vi "DriveSplinePathPlanner.vi"(3 "error in (no error)":errorcluster, 4 "DrivePathPlanParams":T2={"max_velocity (in/s)"=72.0, "max_acceleration (in/s^2)"=20.0, "max_jerk (in/s^3)"=60.0, "dt(ms)"=10, "sample_count"=1000, "wheelbase_width (in)"=24.0} {"dt(ms)" items=["TrajectoryDuration_0ms"=0, "TrajectoryDuration_5ms"=5, "TrajectoryDuration_10ms"=10, "TrajectoryDuration_20ms"=20, "TrajectoryDuration_30ms"=30, "TrajectoryDuration_40ms"=40, "TrajectoryDuration_50ms"=50, "TrajectoryDuration_100ms"=100]}, 5 "path":T5[](array[typedef])=[{"x"=12.0, "y"=150.0, "angle"=0.0}, {"x"=24.0, "y"=150.0, "angle"=0.0}, {"x"=175.0, "y"=275.0, "angle"=0.0}, {"x"=235.0, "y"=200.0, "angle"=90.0}, {"x"=235.0, "y"=125.0, "angle"=90.0}, {"x"=290.0, "y"=65.0, "angle"=0.0}]) -> (0 "error out":errorcluster, 1 "RightTrajectory":T1[](array[typedef]), 2 "LeftTrajectory":T1[](array[typedef]))   [LabVIEW 2017]
uses:
  Pathfinder/Pathfinder-LabVIEW/Pathfinder-Lib/VIs/Waypoint.ctl
  PathPlannerSupport/TypeDefs/DrivePathfinderParams.ctl
  <vilib>/Rock Robotics/WPI/ThirdParty/Phoenix-LabVIEW/Motor Controller/Controls/CTRE_Phoenix_MotorControl_TrajectoryPointTimeDur.ctl
  Pathfinder/Pathfinder-LabVIEW/Pathfinder-Lib/VIs/Segment.ctl
  Pathfinder/Pathfinder-LabVIEW/Pathfinder-Lib/Pathfinder.lvlib
panel:
  in  "Tab Control":enum32{"Primary Path", "Tank Position"}(tab)
  out "Path":T4(graph)=[{"position"=2.9411764705882357e-05, "velocity"=0.005882352941176471, "acceleration"=0.5882352941176471, "jerk"=58.82352941176471, "heading"=0.0}, {"position"=0.00014705882352941178, "velocity"=0.01764705882352941, "acceleration"=1.1764705882352942, "jerk"=58.82352941176471, "heading"=0.0}, {"position"=0.0004117647058823529, "velocity"=0.03529411764705882, "acceleration"=1.7647058823529411, "jerk"=58.823529411764696, "heading"=0.0}, {"position"=0.0008823529411764706, "velocity"=0.0588235294117647, "acceleration"=2.3529411764705874, "jerk"=58.82352941176463, "heading"=0.0}, {"position"=0.0016176470588235292, "velocity"=0.08823529411764705, "acceleration"=2.941176470588235, "jerk"=58.82352941176476, "heading"=0.0}, {"position"=0.002676470588235294, "velocity"=0.12352941176470589, "acceleration"=3.5294117647058836, "jerk"=58.82352941176485, "heading"=0.0}, {"position"=0.00411764705882353, "velocity"=0.16470588235294117, "acceleration"=4.117647058823529, "jerk"=58.82352941176454, "heading"=0.0}, {"position"=0.006, "velocity"=0.21176470588235294, "acceleration"=4.705882352941177, "jerk"=58.82352941176476, "heading"=0.0}, {"position"=0.008382352941176471, "velocity"=0.2647058823529412, "acceleration"=5.294117647058824, "jerk"=58.82352941176476, "heading"=0.0}, {"position"=0.011323529411764706, "velocity"=0.3235294117647059, "acceleration"=5.882352941176472, "jerk"=58.82352941176476, "heading"=0.0}, {"position"=0.014882352941176472, "velocity"=0.38823529411764707, "acceleration"=6.470588235294117, "jerk"=58.8235294117645, "heading"=0.0}, {"position"=0.01911764705882353, "velocity"=0.4588235294117647, "acceleration"=7.058823529411762, "jerk"=58.8235294117645, "heading"=0.0}, {"position"=0.02408823529411765, "velocity"=0.5352941176470588, "acceleration"=7.647058823529412, "jerk"=58.82352941176503, "heading"=0.0}, {"position"=0.02985294117647059, "velocity"=0.6176470588235294, "acceleration"=8.235294117647063, "jerk"=58.823529411765115, "heading"=0.0}, {"position"=0.036470588235294116, "velocity"=0.7058823529411764, "acceleration"=8.823529411764696, "jerk"=58.82352941176325, "heading"=0.0}, {"position"=0.044, "velocity"=0.8, "acceleration"=9.411764705882364, "jerk"=58.823529411766806, "heading"=0.0}, {"position"=0.0525, "velocity"=0.8999999999999999, "acceleration"=9.999999999999986, "jerk"=58.82352941176219, "heading"=0.0}, {"position"=0.06202941176470588, "velocity"=1.0058823529411764, "acceleration"=10.588235294117654, "jerk"=58.823529411766806, "heading"=0.0}, {"position"=0.07264705882352941, "velocity"=1.1176470588235294, "acceleration"=11.176470588235299, "jerk"=58.8235294117645, "heading"=0.0}, {"position"=0.08441176470588235, "velocity"=1.2352941176470589, "acceleration"=11.764705882352944, "jerk"=58.8235294117645, "heading"=0.0}, {"position"=0.09738235294117648, "velocity"=1.3588235294117648, "acceleration"=12.352941176470589, "jerk"=58.8235294117645, "heading"=0.0}, {"position"=0.11161764705882353, "velocity"=1.488235294117647, "acceleration"=12.941176470588234, "jerk"=58.8235294117645, "heading"=0.0}, {"position"=0.1271764705882353, "velocity"=1.623529411764706, "acceleration"=13.5294117647059, "jerk"=58.82352941176663, "heading"=0.0}, {"position"=0.14411764705882354, "velocity"=1.7647058823529411, "acceleration"=14.1176470588235, "jerk"=58.823529411760056, "heading"=0.0}, {"position"=0.1625, "velocity"=1.9117647058823528, "acceleration"=14.705882352941169, "jerk"=58.823529411766806, "heading"=0.0}, {"position"=0.18238235294117647, "velocity"=2.064705882352941, "acceleration"=15.294117647058814, "jerk"=58.8235294117645, "heading"=0.0}, {"position"=0.2038235294117647, "velocity"=2.223529411764706, "acceleration"=15.882352941176503, "jerk"=58.82352941176894, "heading"=0.0}, {"position"=0.22688235294117648, "velocity"=2.388235294117647, "acceleration"=16.4705882352941, "jerk"=58.82352941175988, "heading"=0.0}, {"position"=0.25161764705882356, "velocity"=2.5588235294117645, "acceleration"=17.058823529411747, "jerk"=58.8235294117645, "heading"=0.0}, {"position"=0.2780882352941177, "velocity"=2.735294117647059, "acceleration"=17.647058823529438, "jerk"=58.823529411769115, "heading"=0.0}, {"position"=0.3063529411764706, "velocity"=2.9176470588235297, "acceleration"=18.235294117647083, "jerk"=58.8235294117645, "heading"=0.0}, {"position"=0.33647058823529413, "velocity"=3.1058823529411765, "acceleration"=18.82352941176468, "jerk"=58.82352941175988, "heading"=0.0}, {"position"=0.3685, "velocity"=3.3000000000000003, "acceleration"=19.411764705882373, "jerk"=58.823529411769115, "heading"=0.0}, {"position"=0.40249999999999997, "velocity"=3.4999999999999996, "acceleration"=19.99999999999993, "jerk"=58.823529411755615, "heading"=0.0}, {"position"=0.43849999999999995, "velocity"=3.6999999999999997, "acceleration"=20.000000000000018, "jerk"=8.881784197001252e-12, "heading"=0.0}, {"position"=0.4764999999999999, "velocity"=3.8999999999999995, "acceleration"=19.99999999999997, "jerk"=-4.618527782440651e-12, "heading"=0.0}, {"position"=0.5165, "velocity"=4.1, "acceleration"=20.000000000000018, "jerk"=4.618527782440651e-12, "heading"=0.0}, {"position"=0.5585, "velocity"=4.3, "acceleration"=20.000000000000018, "jerk"=0.0, "heading"=0.0}, {"position"=0.6025, "velocity"=4.5, "acceleration"=20.000000000000018, "jerk"=0.0, "heading"=0.0}, {"position"=0.6485000000000001, "velocity"=4.7, "acceleration"=20.000000000000018, "jerk"=0.0, "heading"=0.0}, {"position"=0.6965000000000001, "velocity"=4.9, "acceleration"=20.000000000000018, "jerk"=0.0, "heading"=0.0}, {"position"=0.7465000000000002, "velocity"=5.1, "acceleration"=19.99999999999993, "jerk"=-8.881784197001252e-12, "heading"=0.0}, {"position"=0.7985000000000002, "velocity"=5.3, "acceleration"=20.000000000000018, "jerk"=8.881784197001252e-12, "heading"=0.0}, {"position"=0.8525000000000003, "velocity"=5.5, "acceleration"=20.000000000000018, "jerk"=0.0, "heading"=0.0}, {"position"=0.9085000000000003, "velocity"=5.700000000000001, "acceleration"=20.000000000000107, "jerk"=8.881784197001252e-12, "heading"=0.0}, {"position"=0.9665000000000004, "velocity"=5.9, "acceleration"=19.99999999999993, "jerk"=-1.7763568394002505e-11, "heading"=0.0}, {"position"=1.0265000000000004, "velocity"=6.1000000000000005, "acceleration"=20.000000000000018, "jerk"=8.881784197001252e-12, "heading"=0.0}, {"position"=1.0885000000000005, "velocity"=6.300000000000001, "acceleration"=20.000000000000018, "jerk"=0.0, "heading"=0.0}, {"position"=1.1525000000000005, "velocity"=6.500000000000001, "acceleration"=20.000000000000018, "jerk"=0.0, "heading"=0.0}, {"position"=1.2185000000000006, "velocity"=6.7, "acceleration"=19.99999999999993, "jerk"=-8.881784197001252e-12, "heading"=0.0}, {"position"=1.2865000000000006, "velocity"=6.8999999999999995, "acceleration"=19.99999999999993, "jerk"=0.0, "heading"=0.0}, {"position"=1.3565000000000007, "velocity"=7.1, "acceleration"=20.000000000000018, "jerk"=8.881784197001252e-12, "heading"=0.0}, {"position"=1.4285000000000008, "velocity"=7.3, "acceleration"=20.000000000000018, "jerk"=0.0, "heading"=0.0}, {"position"=1.5025000000000008, "velocity"=7.499999999999999, "acceleration"=19.99999999999993, "jerk"=-8.881784197001252e-12, "heading"=0.0}, {"position"=1.578500000000001, "velocity"=7.699999999999999, "acceleration"=20.000000000000018, "jerk"=8.881784197001252e-12, "heading"=0.0}, {"position"=1.656500000000001, "velocity"=7.9, "acceleration"=20.000000000000107, "jerk"=8.881784197001252e-12, "heading"=0.0}, {"position"=1.736500000000001, "velocity"=8.1, "acceleration"=19.99999999999993, "jerk"=-1.7763568394002505e-11, "heading"=0.0}, {"position"=1.8185000000000011, "velocity"=8.299999999999999, "acceleration"=19.99999999999993, "jerk"=0.0, "heading"=0.0}, {"position"=1.9025000000000012, "velocity"=8.5, "acceleration"=20.000000000000107, "jerk"=1.7763568394002505e-11, "heading"=0.0}, {"position"=1.9885000000000013, "velocity"=8.7, "acceleration"=19.99999999999993, "jerk"=-1.7763568394002505e-11, "heading"=0.0}, {"position"=2.076500000000001, "velocity"=8.899999999999999, "acceleration"=19.99999999999993, "jerk"=0.0, "heading"=0.0}, {"position"=2.166500000000001, "velocity"=9.1, "acceleration"=20.000000000000107, "jerk"=1.7763568394002505e-11, "heading"=0.0}, {"position"=2.258500000000001, "velocity"=9.299999999999999, "acceleration"=19.99999999999993, "jerk"=-1.7763568394002505e-11, "heading"=0.0}, {"position"=2.352500000000001, "velocity"=9.499999999999998, "acceleration"=19.99999999999993, "jerk"=0.0, "heading"=0.0}, {"position"=2.448500000000001, "velocity"=9.7, "acceleration"=20.000000000000107, "jerk"=1.7763568394002505e-11, "heading"=0.0}, {"position"=2.546500000000001, "velocity"=9.899999999999999, "acceleration"=19.99999999999993, "jerk"=-1.7763568394002505e-11, "heading"=0.0}, {"position"=2.646500000000001, "velocity"=10.1, "acceleration"=20.000000000000107, "jerk"=1.7763568394002505e-11, "heading"=0.0}, {"position"=2.748500000000001, "velocity"=10.299999999999999, "acceleration"=19.99999999999993, "jerk"=-1.7763568394002505e-11, "heading"=0.0}, {"position"=2.852500000000001, "velocity"=10.499999999999998, "acceleration"=19.99999999999993, "jerk"=0.0, "heading"=0.0}, {"position"=2.958500000000001, "velocity"=10.7, "acceleration"=20.000000000000107, "jerk"=1.7763568394002505e-11, "heading"=0.0}, {"position"=3.066500000000001, "velocity"=10.899999999999999, "acceleration"=19.99999999999993, "jerk"=-1.7763568394002505e-11, "heading"=0.0}, {"position"=3.1765000000000008, "velocity"=11.099999999999998, "acceleration"=19.99999999999993, "jerk"=0.0, "heading"=0.0}, {"position"=3.288500000000001, "velocity"=11.3, "acceleration"=20.000000000000284, "jerk"=3.552713678800501e-11, "heading"=0.0}, {"position"=3.4025000000000007, "velocity"=11.5, "acceleration"=19.99999999999993, "jerk"=-3.552713678800501e-11, "heading"=0.0}, {"position"=3.518500000000001, "velocity"=11.700000000000001, "acceleration"=20.000000000000107, "jerk"=1.7763568394002505e-11, "heading"=0.0}, {"position"=3.6365000000000007, "velocity"=11.9, "acceleration"=19.99999999999993, "jerk"=-1.7763568394002505e-11, "heading"=0.0}, {"position"=3.756500000000001, "velocity"=12.1, "acceleration"=19.99999999999993, "jerk"=0.0, "heading"=0.0}, {"position"=3.8785000000000007, "velocity"=12.3, "acceleration"=20.000000000000107, "jerk"=1.7763568394002505e-11, "heading"=0.0}, {"position"=4.0025, "velocity"=12.5, "acceleration"=19.99999999999993, "jerk"=-1.7763568394002505e-11, "heading"=0.0}, {"position"=4.128500000000001, "velocity"=12.7, "acceleration"=19.99999999999993, "jerk"=0.0, "heading"=0.0}, {"position"=4.256500000000001, "velocity"=12.9, "acceleration"=20.000000000000107, "jerk"=1.7763568394002505e-11, "heading"=0.0}, {"position"=4.386500000000001, "velocity"=13.1, "acceleration"=19.99999999999993, "jerk"=-1.7763568394002505e-11, "heading"=0.0}, {"position"=4.5185, "velocity"=13.3, "acceleration"=20.000000000000107, "jerk"=1.7763568394002505e-11, "heading"=0.0}, {"position"=4.652500000000001, "velocity"=13.5, "acceleration"=19.99999999999993, "jerk"=-1.7763568394002505e-11, "heading"=0.0}, {"position"=4.788500000000001, "velocity"=13.7, "acceleration"=19.99999999999993, "jerk"=0.0, "heading"=0.0}, {"position"=4.926500000000001, "velocity"=13.9, "acceleration"=20.000000000000107, "jerk"=1.7763568394002505e-11, "heading"=0.0}, {"position"=5.0665000000000004, "velocity"=14.1, "acceleration"=19.99999999999993, "jerk"=-1.7763568394002505e-11, "heading"=0.0}, {"position"=5.208500000000001, "velocity"=14.3, "acceleration"=20.000000000000107, "jerk"=1.7763568394002505e-11, "heading"=0.0}, {"position"=5.352500000000001, "velocity"=14.5, "acceleration"=19.99999999999993, "jerk"=-1.7763568394002505e-11, "heading"=0.0}, {"position"=5.498500000000001, "velocity"=14.7, "acceleration"=19.99999999999993, "jerk"=0.0, "heading"=0.0}, {"position"=5.6465000000000005, "velocity"=14.9, "acceleration"=20.000000000000107, "jerk"=1.7763568394002505e-11, "heading"=0.0}, {"position"=5.796500000000001, "velocity"=15.1, "acceleration"=19.99999999999993, "jerk"=-1.7763568394002505e-11, "heading"=0.0}, {"position"=5.948500000000001, "velocity"=15.299999999999999, "acceleration"=19.99999999999993, "jerk"=0.0, "heading"=0.0}, {"position"=6.102500000000001, "velocity"=15.5, "acceleration"=20.000000000000107, "jerk"=1.7763568394002505e-11, "heading"=0.0}, {"position"=6.258500000000001, "velocity"=15.7, "acceleration"=19.99999999999993, "jerk"=-1.7763568394002505e-11, "heading"=0.0}, {"position"=6.416500000000001, "velocity"=15.900000000000002, "acceleration"=20.000000000000284, "jerk"=3.552713678800501e-11, "heading"=0.0}, {"position"=6.576500000000001, "velocity"=16.1, "acceleration"=19.99999999999993, "jerk"=-3.552713678800501e-11, "heading"=0.0}, {"position"=6.738500000000001, "velocity"=16.3, "acceleration"=19.99999999999993, "jerk"=0.0, "heading"=0.0}, {"position"=6.902500000000001, "velocity"=16.5, "acceleration"=19.99999999999993, "jerk"=0.0, "heading"=0.0}, {"position"=7.068500000000001, "velocity"=16.7, "acceleration"=19.99999999999993, "jerk"=0.0, "heading"=0.0}, {"position"=7.236500000000001, "velocity"=16.9, "acceleration"=19.99999999999993, "jerk"=0.0, "heading"=0.0}, {"position"=7.406500000000001, "velocity"=17.099999999999998, "acceleration"=19.99999999999993, "jerk"=0.0, "heading"=0.0}, {"position"=7.578500000000001, "velocity"=17.3, "acceleration"=20.000000000000284, "jerk"=3.552713678800501e-11, "heading"=0.0}, {"position"=7.752500000000001, "velocity"=17.5, "acceleration"=19.99999999999993, "jerk"=-3.552713678800501e-11, "heading"=0.0}, {"position"=7.928500000000001, "velocity"=17.7, "acceleration"=19.99999999999993, "jerk"=0.0, "heading"=0.0}, {"position"=8.106500000000002, "velocity"=17.9, "acceleration"=19.99999999999993, "jerk"=0.0, "heading"=0.0}, {"position"=8.286500000000002, "velocity"=18.1, "acceleration"=20.000000000000284, "jerk"=3.552713678800501e-11, "heading"=0.0}, {"position"=8.468500000000002, "velocity"=18.300000000000004, "acceleration"=20.000000000000284, "jerk"=0.0, "heading"=0.0}, {"position"=8.652500000000002, "velocity"=18.5, "acceleration"=19.999999999999574, "jerk"=-7.105427357601002e-11, "heading"=0.0}, {"position"=8.838500000000002, "velocity"=18.700000000000003, "acceleration"=20.000000000000284, "jerk"=7.105427357601002e-11, "heading"=0.0}, {"position"=9.026500000000002, "velocity"=18.900000000000002, "acceleration"=19.99999999999993, "jerk"=-3.552713678800501e-11, "heading"=0.0}, {"position"=9.216500000000002, "velocity"=19.1, "acceleration"=19.99999999999993, "jerk"=0.0, "heading"=0.0}, {"position"=9.408500000000002, "velocity"=19.3, "acceleration"=19.99999999999993, "jerk"=0.0, "heading"=0.0}, {"position"=9.602500000000003, "velocity"=19.500000000000004, "acceleration"=20.000000000000284, "jerk"=3.552713678800501e-11, "heading"=0.0}, {"position"=9.798500000000002, "velocity"=19.7, "acceleration"=19.999999999999574, "jerk"=-7.105427357601002e-11, "heading"=0.0}, {"position"=9.996500000000003, "velocity"=19.900000000000002, "acceleration"=20.000000000000284, "jerk"=7.105427357601002e-11, "heading"=0.0}, {"position"=10.196500000000002, "velocity"=20.1, "acceleration"=19.99999999999993, "jerk"=-3.552713678800501e-11, "heading"=0.0}, {"position"=10.398500000000002, "velocity"=20.3, "acceleration"=19.99999999999993, "jerk"=0.0, "heading"=0.0}, {"position"=10.602500000000003, "velocity"=20.5, "acceleration"=19.99999999999993, "jerk"=0.0, "heading"=0.0}, {"position"=10.808500000000002, "velocity"=20.700000000000003, "acceleration"=20.000000000000284, "jerk"=3.552713678800501e-11, "heading"=0.0}, {"position"=11.016500000000002, "velocity"=20.9, "acceleration"=19.999999999999574, "jerk"=-7.105427357601002e-11, "heading"=0.0}, {"position"=11.226500000000003, "velocity"=21.1, "acceleration"=20.000000000000284, "jerk"=7.105427357601002e-11, "heading"=0.0}, {"position"=11.438500000000003, "velocity"=21.3, "acceleration"=19.99999999999993, "jerk"=-3.552713678800501e-11, "heading"=0.0}, {"position"=11.652500000000003, "velocity"=21.500000000000004, "acceleration"=20.000000000000284, "jerk"=3.552713678800501e-11, "heading"=0.0}, {"position"=11.868500000000003, "velocity"=21.7, "acceleration"=19.999999999999574, "jerk"=-7.105427357601002e-11, "heading"=0.0}, {"position"=12.086500000000003, "velocity"=21.900000000000002, "acceleration"=20.000000000000284, "jerk"=7.105427357601002e-11, "heading"=359.8806943068728}, {"position"=12.306500000000003, "velocity"=22.1, "acceleration"=19.99999999999993, "jerk"=-3.552713678800501e-11, "heading"=0.026596597273722586}, {"position"=12.528500000000003, "velocity"=22.3, "acceleration"=19.99999999999993, "jerk"=0.0, "heading"=0.1743535565500996}, {"position"=12.752500000000003, "velocity"=22.5, "acceleration"=19.99999999999993, "jerk"=0.0, "heading"=0.32416768747403213}, {"position"=12.978500000000004, "velocity"=22.7, "acceleration"=19.99999999999993, "jerk"=0.0, "heading"=0.47603410075499847}, {"position"=13.206500000000004, "velocity"=22.9, "acceleration"=19.99999999999993, "jerk"=0.0, "heading"=0.6299618295768361}, {"position"=13.436500000000004, "velocity"=23.099999999999998, "acceleration"=19.99999999999993, "jerk"=0.0, "heading"=0.7859727327629965}, {"position"=13.668500000000003, "velocity"=23.3, "acceleration"=20.000000000000284, "jerk"=3.552713678800501e-11, "heading"=0.9440887403185972}, {"position"=13.902500000000003, "velocity"=23.499999999999996, "acceleration"=19.999999999999574, "jerk"=-7.105427357601002e-11, "heading"=1.1043318455056377}, {"position"=14.138500000000004, "velocity"=23.7, "acceleration"=20.000000000000284, "jerk"=7.105427357601002e-11, "heading"=1.2667240964869242}, {"position"=14.376500000000004, "velocity"=23.9, "acceleration"=19.99999999999993, "jerk"=-3.552713678800501e-11, "heading"=1.4312875875241853}, {"position"=14.616500000000004, "velocity"=24.1, "acceleration"=20.000000000000284, "jerk"=3.552713678800501e-11, "heading"=1.5980444497155757}, {"position"=14.858500000000003, "velocity"=24.299999999999997, "acceleration"=19.999999999999574, "jerk"=-7.105427357601002e-11, "heading"=1.7670168412578064}, {"position"=15.102500000000003, "velocity"=24.5, "acceleration"=20.000000000000284, "jerk"=7.105427357601002e-11, "heading"=1.938226937217854}, {"position"=15.348500000000003, "velocity"=24.7, "acceleration"=19.99999999999993, "jerk"=-3.552713678800501e-11, "heading"=2.111696918798984}, {"position"=15.596500000000002, "velocity"=24.9, "acceleration"=19.99999999999993, "jerk"=0.0, "heading"=2.2874489620858793}, {"position"=15.846500000000002, "velocity"=25.099999999999998, "acceleration"=19.99999999999993, "jerk"=0.0, "heading"=2.4655052262535966}, {"position"=16.0985, "velocity"=25.3, "acceleration"=20.000000000000284, "jerk"=3.552713678800501e-11, "heading"=2.6458878412247393}, {"position"=16.352500000000003, "velocity"=25.499999999999996, "acceleration"=19.999999999999574, "jerk"=-7.105427357601002e-11, "heading"=2.8286188947596687}, {"position"=16.608500000000003, "velocity"=25.7, "acceleration"=20.000000000000284, "jerk"=7.105427357601002e-11, "heading"=3.0137204189641817}, {"position"=16.866500000000002, "velocity"=25.9, "acceleration"=19.99999999999993, "jerk"=-3.552713678800501e-11, "heading"=3.2012143761994194}, {"position"=17.126500000000004, "velocity"=26.099999999999998, "acceleration"=19.99999999999993, "jerk"=0.0, "heading"=3.391122644378866}, {"position"=17.388500000000004, "velocity"=26.299999999999997, "acceleration"=19.99999999999993, "jerk"=0.0, "heading"=3.5834670016371466}, {"position"=17.652500000000003, "velocity"=26.5, "acceleration"=20.000000000000284, "jerk"=3.552713678800501e-11, "heading"=3.7782691103560753}, {"position"=17.9185, "velocity"=26.699999999999996, "acceleration"=19.999999999999574, "jerk"=-7.105427357601002e-11, "heading"=3.975550500533184}, {"position"=18.186500000000002, "velocity"=26.9, "acceleration"=20.000000000000284, "jerk"=7.105427357601002e-11, "heading"=4.175332552478496}, {"position"=18.456500000000002, "velocity"=27.1, "acceleration"=20.000000000000284, "jerk"=0.0, "heading"=4.377658335678091}, {"position"=18.7285, "velocity"=27.300000000000004, "acceleration"=20.000000000000284, "jerk"=0.0, "heading"=4.582559037811216}, {"position"=19.0025, "velocity"=27.5, "acceleration"=19.999999999999574, "jerk"=-7.105427357601002e-11, "heading"=4.7900277371429345}, {"position"=19.2785, "velocity"=27.700000000000003, "acceleration"=20.000000000000284, "jerk"=7.105427357601002e-11, "heading"=5.000085015447648}, {"position"=19.5565, "velocity"=27.900000000000002, "acceleration"=19.99999999999993, "jerk"=-3.552713678800501e-11, "heading"=5.212751205515084}, {"position"=19.8365, "velocity"=28.1, "acceleration"=19.99999999999993, "jerk"=0.0, "heading"=5.4280463694673555}, {"position"=20.1185, "velocity"=28.3, "acceleration"=19.99999999999993, "jerk"=0.0, "heading"=5.6460030928801945}, {"position"=20.4025, "velocity"=28.500000000000004, "acceleration"=20.000000000000284, "jerk"=3.552713678800501e-11, "heading"=5.8666951092504585}, {"position"=20.6885, "velocity"=28.7, "acceleration"=19.999999999999574, "jerk"=-7.105427357601002e-11, "heading"=6.090078601289142}, {"position"=20.9765, "velocity"=28.900000000000002, "acceleration"=20.000000000000284, "jerk"=7.105427357601002e-11, "heading"=6.316172288510728}, {"position"=21.2665, "velocity"=29.1, "acceleration"=19.99999999999993, "jerk"=-3.552713678800501e-11, "heading"=6.544994497114298}, {"position"=21.558500000000002, "velocity"=29.3, "acceleration"=19.99999999999993, "jerk"=0.0, "heading"=6.776626967962871}, {"position"=21.852500000000003, "velocity"=29.5, "acceleration"=19.99999999999993, "jerk"=0.0, "heading"=7.011060610678886}, {"position"=22.148500000000002, "velocity"=29.700000000000003, "acceleration"=20.000000000000284, "jerk"=3.552713678800501e-11, "heading"=7.2482791275116325}, {"position"=22.4465, "velocity"=29.9, "acceleration"=19.999999999999574, "jerk"=-7.105427357601002e-11, "heading"=7.488298956712767}, {"position"=22.7465, "velocity"=30.1, "acceleration"=20.000000000000284, "jerk"=7.105427357601002e-11, "heading"=7.731244180558999}, {"position"=23.0485, "velocity"=30.3, "acceleration"=19.99999999999993, "jerk"=-3.552713678800501e-11, "heading"=7.977031343589307}, {"position"=23.3525, "velocity"=30.500000000000004, "acceleration"=20.000000000000284, "jerk"=3.552713678800501e-11, "heading"=8.225669605162418}, {"position"=23.6585, "velocity"=30.7, "acceleration"=19.999999999999574, "jerk"=-7.105427357601002e-11, "heading"=8.477266887465865}, {"position"=23.9665, "velocity"=30.900000000000002, "acceleration"=20.000000000000284, "jerk"=7.105427357601002e-11, "heading"=8.731778411856856}, {"position"=24.2765, "velocity"=31.1, "acceleration"=19.99999999999993, "jerk"=-3.552713678800501e-11, "heading"=8.989184788022522}, {"position"=24.5885, "velocity"=31.3, "acceleration"=19.99999999999993, "jerk"=0.0, "heading"=9.249618754216776}, {"position"=24.9025, "velocity"=31.5, "acceleration"=19.99999999999993, "jerk"=0.0, "heading"=9.512990755357727}, {"position"=25.2185, "velocity"=31.7, "acceleration"=19.99999999999993, "jerk"=0.0, "heading"=9.779333344060724}, {"position"=25.5365, "velocity"=31.9, "acceleration"=19.99999999999993, "jerk"=0.0, "heading"=10.04872645588668}, {"position"=25.8565, "velocity"=32.099999999999994, "acceleration"=19.999999999999574, "jerk"=-3.552713678800501e-11, "heading"=10.321072266152298}, {"position"=26.1785, "velocity"=32.300000000000004, "acceleration"=20.000000000000995, "jerk"=1.4210854715202004e-10, "heading"=10.596511622153107}, {"position"=26.5025, "velocity"=32.5, "acceleration"=19.999999999999574, "jerk"=-1.4210854715202004e-10, "heading"=10.874943221246617}, {"position"=26.828500000000002, "velocity"=32.7, "acceleration"=20.000000000000284, "jerk"=7.105427357601002e-11, "heading"=11.156448636107202}, {"position"=27.1565, "velocity"=32.9, "acceleration"=19.999999999999574, "jerk"=-7.105427357601002e-11, "heading"=11.441000593572353}, {"position"=27.4865, "velocity"=33.1, "acceleration"=20.000000000000284, "jerk"=7.105427357601002e-11, "heading"=11.728620941270538}, {"position"=27.8185, "velocity"=33.3, "acceleration"=19.999999999999574, "jerk"=-7.105427357601002e-11, "heading"=12.01931808423193}, {"position"=28.1525, "velocity"=33.5, "acceleration"=20.000000000000284, "jerk"=7.105427357601002e-11, "heading"=12.313091420823161}, {"position"=28.4885, "velocity"=33.7, "acceleration"=20.000000000000284, "jerk"=0.0, "heading"=12.609948057440935}, {"position"=28.8265, "velocity"=33.9, "acceleration"=19.999999999999574, "jerk"=-7.105427357601002e-11, "heading"=12.909900751455448}, {"position"=29.1665, "velocity"=34.1, "acceleration"=20.000000000000284, "jerk"=7.105427357601002e-11, "heading"=13.212919886317012}, {"position"=29.508499999999998, "velocity"=34.300000000000004, "acceleration"=20.000000000000284, "jerk"=0.0, "heading"=13.519065744339041}, {"position"=29.8525, "velocity"=34.5, "acceleration"=19.999999999999574, "jerk"=-7.105427357601002e-11, "heading"=13.828240486659336}, {"position"=30.1985, "velocity"=34.7, "acceleration"=20.000000000000284, "jerk"=7.105427357601002e-11, "heading"=14.140577686116911}, {"position"=30.546499999999998, "velocity"=34.9, "acceleration"=19.999999999999574, "jerk"=-7.105427357601002e-11, "heading"=14.455946107562308}, {"position"=30.8965, "velocity"=35.1, "acceleration"=20.000000000000284, "jerk"=7.105427357601002e-11, "heading"=14.774400694365548}, {"position"=31.2485, "velocity"=35.3, "acceleration"=19.999999999999574, "jerk"=-7.105427357601002e-11, "heading"=15.095941142291279}, {"position"=31.6025, "velocity"=35.5, "acceleration"=20.000000000000284, "jerk"=7.105427357601002e-11, "heading"=15.420499989261904}, {"position"=31.9585, "velocity"=35.7, "acceleration"=20.000000000000284, "jerk"=0.0, "heading"=15.74814535080236}, {"position"=32.3165, "velocity"=35.900000000000006, "acceleration"=20.000000000000284, "jerk"=0.0, "heading"=16.07881887293392}, {"position"=32.6765, "velocity"=36.1, "acceleration"=19.999999999999574, "jerk"=-7.105427357601002e-11, "heading"=16.412480925063015}, {"position"=33.0385, "velocity"=36.3, "acceleration"=19.999999999999574, "jerk"=0.0, "heading"=16.749173156086542}, {"position"=33.402499999999996, "velocity"=36.5, "acceleration"=20.000000000000284, "jerk"=7.105427357601002e-11, "heading"=17.088853886892473}, {"position"=33.768499999999996, "velocity"=36.699999999999996, "acceleration"=19.999999999999574, "jerk"=-7.105427357601002e-11, "heading"=17.43147260999384}, {"position"=34.1365, "velocity"=36.900000000000006, "acceleration"=20.000000000000995, "jerk"=1.4210854715202004e-10, "heading"=17.777011519354833}, {"position"=34.506499999999996, "velocity"=37.1, "acceleration"=19.999999999999574, "jerk"=-1.4210854715202004e-10, "heading"=18.12551174609648}, {"position"=34.878499999999995, "velocity"=37.3, "acceleration"=19.999999999999574, "jerk"=0.0, "heading"=18.476877498216318}, {"position"=35.2525, "velocity"=37.49999999999999, "acceleration"=19.999999999999574, "jerk"=0.0, "heading"=18.831081570371552}, {"position"=35.628499999999995, "velocity"=37.7, "acceleration"=20.000000000000995, "jerk"=1.4210854715202004e-10, "heading"=19.18809404549836}, {"position"=36.006499999999996, "velocity"=37.9, "acceleration"=19.999999999999574, "jerk"=-1.4210854715202004e-10, "heading"=19.54790694135234}, {"position"=36.3865, "velocity"=38.1, "acceleration"=20.000000000000284, "jerk"=7.105427357601002e-11, "heading"=19.910478598411913}, {"position"=36.768499999999996, "velocity"=38.3, "acceleration"=19.999999999999574, "jerk"=-7.105427357601002e-11, "heading"=20.275747054027956}, {"position"=37.152499999999996, "velocity"=38.50000000000001, "acceleration"=20.000000000000995, "jerk"=1.4210854715202004e-10, "heading"=20.643671446851233}, {"position"=37.5385, "velocity"=38.699999999999996, "acceleration"=19.999999999998863, "jerk"=-2.1316282072803006e-10, "heading"=21.01420807888143}, {"position"=37.9265, "velocity"=38.9, "acceleration"=20.000000000000284, "jerk"=1.4210854715202004e-10, "heading"=21.387310403333622}, {"position"=38.3165, "velocity"=39.099999999999994, "acceleration"=19.999999999999574, "jerk"=-7.105427357601002e-11, "heading"=21.762929017795752}, {"position"=38.7085, "velocity"=39.300000000000004, "acceleration"=20.000000000000995, "jerk"=1.4210854715202004e-10, "heading"=22.14102219251801}, {"position"=39.1025, "velocity"=39.5, "acceleration"=19.999999999999574, "jerk"=-1.4210854715202004e-10, "heading"=22.521530504437102}, {"position"=39.4985, "velocity"=39.7, "acceleration"=20.000000000000284, "jerk"=7.105427357601002e-11, "heading"=22.904386067504515}, {"position"=39.8965, "velocity"=39.89999999999999, "acceleration"=19.999999999998863, "jerk"=-1.4210854715202004e-10, "heading"=23.28952833347874}, {"position"=40.2965, "velocity"=40.1, "acceleration"=20.000000000000995, "jerk"=2.1316282072803006e-10, "heading"=23.67689395097623}, {"position"=40.6985, "velocity"=40.3, "acceleration"=19.999999999999574, "jerk"=-1.4210854715202004e-10, "heading"=24.066416792892216}, {"position"=41.102500000000006, "velocity"=40.5, "acceleration"=20.000000000000284, "jerk"=7.105427357601002e-11, "heading"=24.45802798997979}, {"position"=41.508500000000005, "velocity"=40.7, "acceleration"=20.000000000000284, "jerk"=0.0, "heading"=24.851655970631484}, {"position"=41.916500000000006, "velocity"=40.9, "acceleration"=19.999999999999574, "jerk"=-7.105427357601002e-11, "heading"=25.247226506882512}, {"position"=42.3265, "velocity"=41.10000000000001, "acceleration"=20.000000000000995, "jerk"=1.4210854715202004e-10, "heading"=25.6446627666302}, {"position"=42.7385, "velocity"=41.3, "acceleration"=19.999999999998863, "jerk"=-2.1316282072803006e-10, "heading"=26.043885372037998}, {"position"=43.1525, "velocity"=41.5, "acceleration"=20.000000000000284, "jerk"=1.4210854715202004e-10, "heading"=26.444812464065823}, {"position"=43.5685, "velocity"=41.699999999999996, "acceleration"=19.999999999999574, "jerk"=-7.105427357601002e-11, "heading"=26.847359773041763}, {"position"=43.9865, "velocity"=41.900000000000006, "acceleration"=20.000000000000995, "jerk"=1.4210854715202004e-10, "heading"=27.251440695162977}, {"position"=44.4065, "velocity"=42.1, "acceleration"=19.999999999999574, "jerk"=-1.4210854715202004e-10, "heading"=27.65697385589227}, {"position"=44.8285, "velocity"=42.300000000000004, "acceleration"=20.000000000000284, "jerk"=7.105427357601002e-11, "heading"=28.063867292328702}, {"position"=45.2525, "velocity"=42.49999999999999, "acceleration"=19.999999999998863, "jerk"=-1.4210854715202004e-10, "heading"=28.47202190092313}, {"position"=45.6785, "velocity"=42.7, "acceleration"=20.000000000000995, "jerk"=2.1316282072803006e-10, "heading"=28.881342419793967}, {"position"=46.1065, "velocity"=42.9, "acceleration"=19.999999999999574, "jerk"=-1.4210854715202004e-10, "heading"=29.291731725274477}, {"position"=46.5365, "velocity"=43.1, "acceleration"=20.000000000000284, "jerk"=7.105427357601002e-11, "heading"=29.70309094059028}, {"position"=46.9685, "velocity"=43.3, "acceleration"=19.999999999999574, "jerk"=-7.105427357601002e-11, "heading"=30.115319548906836}, {"position"=47.402499999999996, "velocity"=43.50000000000001, "acceleration"=20.000000000000995, "jerk"=1.4210854715202004e-10, "heading"=30.528323395277617}, {"position"=47.838499999999996, "velocity"=43.7, "acceleration"=19.999999999999574, "jerk"=-1.4210854715202004e-10, "heading"=30.942001560280808}, {"position"=48.2765, "velocity"=43.9, "acceleration"=19.999999999999574, "jerk"=0.0, "heading"=31.35623811547934}, {"position"=48.716499999999996, "velocity"=44.099999999999994, "acceleration"=19.999999999999574, "jerk"=0.0, "heading"=31.770927045123866}, {"position"=49.1585, "velocity"=44.300000000000004, "acceleration"=20.000000000000995, "jerk"=1.4210854715202004e-10, "heading"=32.18596132182092}, {"position"=49.6025, "velocity"=44.5, "acceleration"=19.999999999999574, "jerk"=-1.4210854715202004e-10, "heading"=32.601247061400166}, {"position"=50.0485, "velocity"=44.7, "acceleration"=20.000000000000284, "jerk"=7.105427357601002e-11, "heading"=33.016664546918}, {"position"=50.4965, "velocity"=44.9, "acceleration"=19.999999999999574, "jerk"=-7.105427357601002e-11, "heading"=33.43210003784553}, {"position"=50.9465, "velocity"=45.1, "acceleration"=20.000000000000284, "jerk"=7.105427357601002e-11, "heading"=33.84744396115525}, {"position"=51.3985, "velocity"=45.3, "acceleration"=19.999999999999574, "jerk"=-7.105427357601002e-11, "heading"=34.26260148922997}, {"position"=51.8525, "velocity"=45.5, "acceleration"=20.000000000000284, "jerk"=7.105427357601002e-11, "heading"=34.67744480699883}, {"position"=52.3085, "velocity"=45.699999999999996, "acceleration"=19.999999999999574, "jerk"=-7.105427357601002e-11, "heading"=35.09186344190509}, {"position"=52.7665, "velocity"=45.900000000000006, "acceleration"=20.000000000000995, "jerk"=1.4210854715202004e-10, "heading"=35.505757133188844}, {"position"=53.2265, "velocity"=46.1, "acceleration"=19.999999999999574, "jerk"=-1.4210854715202004e-10, "heading"=35.91900678357549}, {"position"=53.688500000000005, "velocity"=46.3, "acceleration"=19.999999999999574, "jerk"=0.0, "heading"=36.33149925046029}, {"position"=54.1525, "velocity"=46.49999999999999, "acceleration"=19.999999999999574, "jerk"=0.0, "heading"=36.74313358060122}, {"position"=54.618500000000004, "velocity"=46.7, "acceleration"=20.000000000000995, "jerk"=1.4210854715202004e-10, "heading"=37.15379197572769}, {"position"=55.0865, "velocity"=46.9, "acceleration"=19.999999999999574, "jerk"=-1.4210854715202004e-10, "heading"=37.56336619227703}, {"position"=55.5565, "velocity"=47.1, "acceleration"=20.000000000000284, "jerk"=7.105427357601002e-11, "heading"=37.971752279120025}, {"position"=56.0285, "velocity"=47.3, "acceleration"=19.999999999999574, "jerk"=-7.105427357601002e-11, "heading"=38.37883730864982}, {"position"=56.5025, "velocity"=47.50000000000001, "acceleration"=20.000000000000995, "jerk"=1.4210854715202004e-10, "heading"=38.784518515793984}, {"position"=56.9785, "velocity"=47.699999999999996, "acceleration"=19.999999999998863, "jerk"=-2.1316282072803006e-10, "heading"=39.18868887655483}, {"position"=57.4565, "velocity"=47.9, "acceleration"=20.000000000000284, "jerk"=1.4210854715202004e-10, "heading"=39.59124477354378}, {"position"=57.936499999999995, "velocity"=48.099999999999994, "acceleration"=19.999999999999574, "jerk"=-7.105427357601002e-11, "heading"=39.9920837075402}, {"position"=58.418499999999995, "velocity"=48.300000000000004, "acceleration"=20.000000000000995, "jerk"=1.4210854715202004e-10, "heading"=40.39110502847616}, {"position"=58.902499999999996, "velocity"=48.5, "acceleration"=19.999999999999574, "jerk"=-1.4210854715202004e-10, "heading"=40.78820768253438}, {"position"=59.38849999999999, "velocity"=48.7, "acceleration"=20.000000000000284, "jerk"=7.105427357601002e-11, "heading"=41.183296941635234}, {"position"=59.87649999999999, "velocity"=48.89999999999999, "acceleration"=19.999999999998863, "jerk"=-1.4210854715202004e-10, "heading"=41.57627203558992}, {"position"=60.366499999999995, "velocity"=49.1, "acceleration"=20.000000000000995, "jerk"=2.1316282072803006e-10, "heading"=41.9670452595938}, {"position"=60.85849999999999, "velocity"=49.3, "acceleration"=19.999999999999574, "jerk"=-1.4210854715202004e-10, "heading"=42.35551654933896}, {"position"=61.35249999999999, "velocity"=49.5, "acceleration"=20.000000000000284, "jerk"=7.105427357601002e-11, "heading"=42.7416047913788}, {"position"=61.848499999999994, "velocity"=49.7, "acceleration"=20.000000000000284, "jerk"=0.0, "heading"=43.12521231746116}, {"position"=62.34649999999999, "velocity"=49.9, "acceleration"=19.999999999999574, "jerk"=-7.105427357601002e-11, "heading"=43.50626294346573}, {"position"=62.84649999999999, "velocity"=50.10000000000001, "acceleration"=20.000000000000995, "jerk"=1.4210854715202004e-10, "heading"=43.88466406028942}, {"position"=63.348499999999994, "velocity"=50.3, "acceleration"=19.999999999998863, "jerk"=-2.1316282072803006e-10, "heading"=44.26034180367996}, {"position"=63.85249999999999, "velocity"=50.5, "acceleration"=20.000000000000284, "jerk"=1.4210854715202004e-10, "heading"=44.63321198855724}, {"position"=64.35849999999999, "velocity"=50.699999999999996, "acceleration"=19.999999999999574, "jerk"=-7.105427357601002e-11, "heading"=45.00319977343231}, {"position"=64.86649999999999, "velocity"=50.900000000000006, "acceleration"=20.000000000000995, "jerk"=1.4210854715202004e-10, "heading"=45.37023321855684}, {"position"=65.3765, "velocity"=51.1, "acceleration"=19.999999999999574, "jerk"=-1.4210854715202004e-10, "heading"=45.7342327555875}, {"position"=65.8885, "velocity"=51.300000000000004, "acceleration"=20.000000000000284, "jerk"=7.105427357601002e-11, "heading"=46.09513977483702}, {"position"=66.40249999999999, "velocity"=51.49999999999999, "acceleration"=19.999999999998863, "jerk"=-1.4210854715202004e-10, "heading"=46.45287491225757}, {"position"=66.9185, "velocity"=51.7, "acceleration"=20.000000000000995, "jerk"=2.1316282072803006e-10, "heading"=46.80738222863207}, {"position"=67.4365, "velocity"=51.9, "acceleration"=19.999999999999574, "jerk"=-1.4210854715202004e-10, "heading"=47.15859901281673}, {"position"=67.95649999999999, "velocity"=52.1, "acceleration"=20.000000000000284, "jerk"=7.105427357601002e-11, "heading"=47.506456423487805}, {"position"=68.4785, "velocity"=52.3, "acceleration"=19.999999999999574, "jerk"=-7.105427357601002e-11, "heading"=47.850908679724334}, {"position"=69.0025, "velocity"=52.50000000000001, "acceleration"=20.000000000000995, "jerk"=1.4210854715202004e-10, "heading"=48.19189294187661}, {"position"=69.5285, "velocity"=52.7, "acceleration"=19.999999999999574, "jerk"=-1.4210854715202004e-10, "heading"=48.52935576717652}, {"position"=70.0565, "velocity"=52.9, "acceleration"=19.999999999999574, "jerk"=0.0, "heading"=48.863254157558934}, {"position"=70.5865, "velocity"=53.099999999999994, "acceleration"=19.999999999999574, "jerk"=0.0, "heading"=49.193530925209316}, {"position"=71.1185, "velocity"=53.300000000000004, "acceleration"=20.000000000000995, "jerk"=1.4210854715202004e-10, "heading"=49.520142390798135}, {"position"=71.6525, "velocity"=53.5, "acceleration"=19.999999999999574, "jerk"=-1.4210854715202004e-10, "heading"=49.84305056767106}, {"position"=72.1885, "velocity"=53.7, "acceleration"=20.000000000000284, "jerk"=7.105427357601002e-11, "heading"=50.162206809702525}, {"position"=72.7265, "velocity"=53.9, "acceleration"=19.999999999999574, "jerk"=-7.105427357601002e-11, "heading"=50.47757084572062}, {"position"=73.26650000000001, "velocity"=54.1, "acceleration"=20.000000000000284, "jerk"=7.105427357601002e-11, "heading"=50.78911219457379}, {"position"=73.80850000000001, "velocity"=54.3, "acceleration"=19.999999999999574, "jerk"=-7.105427357601002e-11, "heading"=51.09679343393174}, {"position"=74.3525, "velocity"=54.5, "acceleration"=20.000000000000284, "jerk"=7.105427357601002e-11, "heading"=51.400571311146905}, {"position"=74.89850000000001, "velocity"=54.699999999999996, "acceleration"=19.999999999999574, "jerk"=-7.105427357601002e-11, "heading"=51.70042528733582}, {"position"=75.44650000000001, "velocity"=54.900000000000006, "acceleration"=20.000000000000995, "jerk"=1.4210854715202004e-10, "heading"=51.99632526765456}, {"position"=75.99650000000001, "velocity"=55.1, "acceleration"=19.999999999999574, "jerk"=-1.4210854715202004e-10, "heading"=52.2882375933615}, {"position"=76.54850000000002, "velocity"=55.3, "acceleration"=19.999999999999574, "jerk"=0.0, "heading"=52.57613532771344}, {"position"=77.10250000000002, "velocity"=55.49999999999999, "acceleration"=19.999999999999574, "jerk"=0.0, "heading"=52.859999714327685}, {"position"=77.65850000000002, "velocity"=55.7, "acceleration"=20.000000000000995, "jerk"=1.4210854715202004e-10, "heading"=53.13980742600156}, {"position"=78.21650000000002, "velocity"=55.9, "acceleration"=19.999999999999574, "jerk"=-1.4210854715202004e-10, "heading"=53.41553256949202}, {"position"=78.77650000000003, "velocity"=56.1, "acceleration"=20.000000000000284, "jerk"=7.105427357601002e-11, "heading"=53.68715368105553}, {"position"=79.33850000000002, "velocity"=56.3, "acceleration"=19.999999999999574, "jerk"=-7.105427357601002e-11, "heading"=53.95465762080504}, {"position"=79.90250000000003, "velocity"=56.50000000000001, "acceleration"=20.000000000000995, "jerk"=1.4210854715202004e-10, "heading"=54.21802680426127}, {"position"=80.46850000000003, "velocity"=56.699999999999996, "acceleration"=19.999999999998863, "jerk"=-2.1316282072803006e-10, "heading"=54.477244912443894}, {"position"=81.03650000000003, "velocity"=56.9, "acceleration"=20.000000000000284, "jerk"=1.4210854715202004e-10, "heading"=54.73229036204334}, {"position"=81.60650000000003, "velocity"=57.099999999999994, "acceleration"=19.999999999999574, "jerk"=-7.105427357601002e-11, "heading"=54.98315491585318}, {"position"=82.17850000000003, "velocity"=57.300000000000004, "acceleration"=20.000000000000995, "jerk"=1.4210854715202004e-10, "heading"=55.22982693600377}, {"position"=82.75250000000003, "velocity"=57.5, "acceleration"=19.999999999999574, "jerk"=-1.4210854715202004e-10, "heading"=55.47229450171895}, {"position"=83.32850000000002, "velocity"=57.7, "acceleration"=20.000000000000284, "jerk"=7.105427357601002e-11, "heading"=55.710546622650085}, {"position"=83.90650000000002, "velocity"=57.89999999999999, "acceleration"=19.999999999998863, "jerk"=-1.4210854715202004e-10, "heading"=55.94457057386897}, {"position"=84.48650000000002, "velocity"=58.1, "acceleration"=20.000000000000995, "jerk"=2.1316282072803006e-10, "heading"=56.174356893930124}, {"position"=85.06850000000001, "velocity"=58.3, "acceleration"=19.999999999999574, "jerk"=-1.4210854715202004e-10, "heading"=56.39990023138972}, {"position"=85.65250000000002, "velocity"=58.5, "acceleration"=20.000000000000284, "jerk"=7.105427357601002e-11, "heading"=56.62119264710238}, {"position"=86.23850000000002, "velocity"=58.7, "acceleration"=20.000000000000284, "jerk"=0.0, "heading"=56.83822680282088}, {"position"=86.82650000000001, "velocity"=58.9, "acceleration"=19.999999999999574, "jerk"=-7.105427357601002e-11, "heading"=57.05099589733922}, {"position"=87.41650000000001, "velocity"=59.10000000000001, "acceleration"=20.000000000000995, "jerk"=1.4210854715202004e-10, "heading"=57.259493603263145}, {"position"=88.00850000000001, "velocity"=59.3, "acceleration"=19.999999999998863, "jerk"=-2.1316282072803006e-10, "heading"=57.463711890450135}, {"position"=88.6025, "velocity"=59.5, "acceleration"=20.000000000000284, "jerk"=1.4210854715202004e-10, "heading"=57.663646367361295}, {"position"=89.19850000000001, "velocity"=59.699999999999996, "acceleration"=19.999999999999574, "jerk"=-7.105427357601002e-11, "heading"=57.859293090037546}, {"position"=89.79650000000001, "velocity"=59.900000000000006, "acceleration"=20.000000000000995, "jerk"=1.4210854715202004e-10, "heading"=58.0506469892967}, {"position"=90.3965, "velocity"=60.1, "acceleration"=19.999999999999574, "jerk"=-1.4210854715202004e-10, "heading"=58.23770316379314}, {"position"=90.9985, "velocity"=60.300000000000004, "acceleration"=20.000000000000284, "jerk"=7.105427357601002e-11, "heading"=58.420456821511074}, {"position"=91.6025, "velocity"=60.49999999999999, "acceleration"=19.999999999998863, "jerk"=-1.4210854715202004e-10, "heading"=58.59890322207649}, {"position"=92.2085, "velocity"=60.7, "acceleration"=20.000000000000995, "jerk"=2.1316282072803006e-10, "heading"=58.77303761988961}, {"position"=92.8165, "velocity"=60.9, "acceleration"=19.999999999999574, "jerk"=-1.4210854715202004e-10, "heading"=58.94285520807504}, {"position"=93.4265, "velocity"=61.1, "acceleration"=20.000000000000284, "jerk"=7.105427357601002e-11, "heading"=59.10835106324084}, {"position"=94.0385, "velocity"=61.3, "acceleration"=19.999999999999574, "jerk"=-7.105427357601002e-11, "heading"=59.269520091033726}, {"position"=94.6525, "velocity"=61.50000000000001, "acceleration"=20.000000000000995, "jerk"=1.4210854715202004e-10, "heading"=59.42635684820294}, {"position"=95.2685, "velocity"=61.7, "acceleration"=19.999999999999574, "jerk"=-1.4210854715202004e-10, "heading"=59.578855258621985}, {"position"=95.8865, "velocity"=61.9, "acceleration"=19.999999999999574, "jerk"=0.0, "heading"=59.72701018403149}, {"position"=96.5065, "velocity"=62.099999999999994, "acceleration"=19.999999999999574, "jerk"=0.0, "heading"=59.870815297798906}, {"position"=97.1285, "velocity"=62.300000000000004, "acceleration"=20.000000000000995, "jerk"=1.4210854715202004e-10, "heading"=60.01026384170946}, {"position"=97.7525, "velocity"=62.5, "acceleration"=19.999999999999574, "jerk"=-1.4210854715202004e-10, "heading"=60.145348575884064}, {"position"=98.3785, "velocity"=62.7, "acceleration"=20.000000000000284, "jerk"=7.105427357601002e-11, "heading"=60.276061729294845}, {"position"=99.0065, "velocity"=62.9, "acceleration"=19.999999999999574, "jerk"=-7.105427357601002e-11, "heading"=60.40239495083989}, {"position"=99.6365, "velocity"=63.1, "acceleration"=20.000000000000284, "jerk"=7.105427357601002e-11, "heading"=60.52433926093727}, {"position"=100.2685, "velocity"=63.3, "acceleration"=19.999999999999574, "jerk"=-7.105427357601002e-11, "heading"=60.641885003596336}, {"position"=100.9025, "velocity"=63.5, "acceleration"=20.000000000000284, "jerk"=7.105427357601002e-11, "heading"=60.755021798923224}, {"position"=101.5385, "velocity"=63.699999999999996, "acceleration"=19.999999999999574, "jerk"=-7.105427357601002e-11, "heading"=60.86373849601625}, {"position"=102.1765, "velocity"=63.900000000000006, "acceleration"=20.000000000000995, "jerk"=1.4210854715202004e-10, "heading"=60.968023126205615}, {"position"=102.8165, "velocity"=64.10000000000001, "acceleration"=20.000000000000284, "jerk"=-7.105427357601002e-11, "heading"=61.06786285659148}, {"position"=103.4585, "velocity"=64.3, "acceleration"=19.999999999998863, "jerk"=-1.4210854715202004e-10, "heading"=61.16324394383369}, {"position"=104.1025, "velocity"=64.5, "acceleration"=20.000000000000284, "jerk"=1.4210854715202004e-10, "heading"=61.25415137640325}, {"position"=104.7485, "velocity"=64.7, "acceleration"=20.000000000000284, "jerk"=0.0, "heading"=61.340569778870275}, {"position"=105.3965, "velocity"=64.9, "acceleration"=20.000000000000284, "jerk"=0.0, "heading"=61.4224824166881}, {"position"=106.04650000000001, "velocity"=65.1, "acceleration"=19.999999999998863, "jerk"=-1.4210854715202004e-10, "heading"=61.49987145240259}, {"position"=106.69850000000001, "velocity"=65.3, "acceleration"=20.000000000000284, "jerk"=1.4210854715202004e-10, "heading"=61.57271790792199}, {"position"=107.3525, "velocity"=65.5, "acceleration"=20.000000000000284, "jerk"=0.0, "heading"=61.64100161878644}, {"position"=108.00850000000001, "velocity"=65.7, "acceleration"=20.000000000000284, "jerk"=0.0, "heading"=61.70470118836346}, {"position"=108.66650000000001, "velocity"=65.89999999999999, "acceleration"=19.999999999998863, "jerk"=-1.4210854715202004e-10, "heading"=61.76379394192538}, {"position"=109.32650000000001, "velocity"=66.1, "acceleration"=20.000000000000284, "jerk"=1.4210854715202004e-10, "heading"=61.81825588056491}, {"position"=109.98850000000002, "velocity"=66.30000000000001, "acceleration"=20.000000000001705, "jerk"=1.4210854715202004e-10, "heading"=61.868061634907505}, {"position"=110.65250000000002, "velocity"=66.5, "acceleration"=19.999999999998863, "jerk"=-2.842170943040401e-10, "heading"=61.91318437441721}, {"position"=111.31850000000001, "velocity"=66.7, "acceleration"=20.000000000000284, "jerk"=1.4210854715202004e-10, "heading"=61.95359579540202}, {"position"=111.98650000000002, "velocity"=66.89999999999999, "acceleration"=19.999999999998863, "jerk"=-1.4210854715202004e-10, "heading"=61.989266296204946}, {"position"=112.65650000000002, "velocity"=67.1, "acceleration"=20.000000000000284, "jerk"=1.4210854715202004e-10, "heading"=62.02016454913396}, {"position"=113.32850000000002, "velocity"=67.3, "acceleration"=20.000000000000284, "jerk"=0.0, "heading"=62.04625761849339}, {"position"=114.00250000000003, "velocity"=67.5, "acceleration"=20.000000000000284, "jerk"=0.0, "heading"=62.067510912261895}, {"position"=114.67850000000003, "velocity"=67.7, "acceleration"=20.000000000000284, "jerk"=0.0, "heading"=62.083888130250266}, {"position"=115.35650000000003, "velocity"=67.9, "acceleration"=20.000000000000284, "jerk"=0.0, "heading"=62.09535121736369}, {"position"=116.03650000000003, "velocity"=68.1, "acceleration"=19.999999999998863, "jerk"=-1.4210854715202004e-10, "heading"=62.10186034212388}, {"position"=116.71850000000003, "velocity"=68.30000000000001, "acceleration"=20.000000000001705, "jerk"=2.842170943040401e-10, "heading"=62.103373775978746}, {"position"=117.40250000000003, "velocity"=68.5, "acceleration"=19.999999999998863, "jerk"=-2.842170943040401e-10, "heading"=62.09984788353514}, {"position"=118.08850000000004, "velocity"=68.7, "acceleration"=20.000000000000284, "jerk"=1.4210854715202004e-10, "heading"=62.091237063169494}, {"position"=118.77647058823533, "velocity"=68.89411764705882, "acceleration"=19.41176470588175, "jerk"=-58.823529411853315, "heading"=62.07749437311427}, {"position"=119.46635294117651, "velocity"=69.08235294117647, "acceleration"=18.82352941176464, "jerk"=-58.823529411711206, "heading"=62.05857261660677}, {"position"=120.15808823529416, "velocity"=69.26470588235294, "acceleration"=18.235294117647527, "jerk"=-58.823529411711206, "heading"=62.03442424658377}, {"position"=120.85161764705886, "velocity"=69.44117647058823, "acceleration"=17.647058823528994, "jerk"=-58.823529411853315, "heading"=62.00500125147322}, {"position"=121.54688235294121, "velocity"=69.61176470588235, "acceleration"=17.05882352941188, "jerk"=-58.823529411711206, "heading"=61.970255182823}, {"position"=122.2438235294118, "velocity"=69.7764705882353, "acceleration"=16.47058823529477, "jerk"=-58.823529411711206, "heading"=61.93013730746935}, {"position"=122.94238235294121, "velocity"=69.93529411764706, "acceleration"=15.882352941176237, "jerk"=-58.823529411853315, "heading"=61.88459835919842}, {"position"=123.64250000000003, "velocity"=70.08823529411765, "acceleration"=15.294117647059124, "jerk"=-58.823529411711206, "heading"=61.83358803530867}, {"position"=124.34411764705885, "velocity"=70.23529411764706, "acceleration"=14.705882352940591, "jerk"=-58.823529411853315, "heading"=61.77705637907407}, {"position"=125.04717647058827, "velocity"=70.37647058823529, "acceleration"=14.11764705882348, "jerk"=-58.823529411711206, "heading"=61.71495259511413}, {"position"=125.75161764705885, "velocity"=70.51176470588236, "acceleration"=13.529411764706367, "jerk"=-58.823529411711206, "heading"=61.64722451387319}, {"position"=126.45738235294121, "velocity"=70.64117647058823, "acceleration"=12.941176470587834, "jerk"=-58.823529411853315, "heading"=61.57382056440788}, {"position"=127.16441176470592, "velocity"=70.76470588235294, "acceleration"=12.352941176470722, "jerk"=-58.823529411711206, "heading"=61.49468845731021}, {"position"=127.87264705882356, "velocity"=70.88235294117646, "acceleration"=11.764705882352189, "jerk"=-58.823529411853315, "heading"=61.409773740526155}, {"position"=128.58202941176472, "velocity"=70.99411764705881, "acceleration"=11.176470588235077, "jerk"=-58.823529411711206, "heading"=61.319023622746485}, {"position"=129.29250000000002, "velocity"=71.10000000000001, "acceleration"=10.588235294119386, "jerk"=-58.8235294115691, "heading"=61.2223839792152}, {"position"=130.00400000000002, "velocity"=71.19999999999999, "acceleration"=9.99999999999801, "jerk"=-58.82352941213753, "heading"=61.11979799103079}, {"position"=130.71647058823532, "velocity"=71.29411764705881, "acceleration"=9.41176470588232, "jerk"=-58.8235294115691, "heading"=61.01121224108017}, {"position"=131.4298529411765, "velocity"=71.38235294117648, "acceleration"=8.823529411766629, "jerk"=-58.8235294115691, "heading"=60.89656952276138}, {"position"=132.14408823529416, "velocity"=71.46470588235293, "acceleration"=8.235294117645253, "jerk"=-58.82352941213753, "heading"=60.77581291851324}, {"position"=132.85911764705887, "velocity"=71.54117647058823, "acceleration"=7.647058823529562, "jerk"=-58.8235294115691, "heading"=60.64888729697189}, {"position"=133.57488235294122, "velocity"=71.61176470588236, "acceleration"=7.058823529413871, "jerk"=-58.8235294115691, "heading"=60.51573143879659}, {"position"=134.2913235294118, "velocity"=71.67647058823529, "acceleration"=6.470588235292496, "jerk"=-58.82352941213753, "heading"=60.376291075159436}, {"position"=135.00838235294123, "velocity"=71.73529411764706, "acceleration"=5.882352941176805, "jerk"=-58.8235294115691, "heading"=60.230505755635235}, {"position"=135.72600000000006, "velocity"=71.78823529411764, "acceleration"=5.294117647058272, "jerk"=-58.823529411853315, "heading"=60.07831717575035}, {"position"=136.44411764705887, "velocity"=71.83529411764707, "acceleration"=4.705882352942581, "jerk"=-58.8235294115691, "heading"=59.91966795889611}, {"position"=137.16267647058828, "velocity"=71.8764705882353, "acceleration"=4.117647058824048, "jerk"=-58.823529411853315, "heading"=59.75449545544221}, {"position"=137.88161764705887, "velocity"=71.91176470588236, "acceleration"=3.5294117647055145, "jerk"=-58.823529411853315, "heading"=59.5827457243077}, {"position"=138.60088235294123, "velocity"=71.94117647058823, "acceleration"=2.9411764705869814, "jerk"=-58.823529411853315, "heading"=59.40435286340221}, {"position"=139.32041176470594, "velocity"=71.96470588235294, "acceleration"=2.3529411764712904, "jerk"=-58.8235294115691, "heading"=59.219264462427105}, {"position"=140.04014705882358, "velocity"=71.98235294117647, "acceleration"=1.7647058823527573, "jerk"=-58.823529411853315, "heading"=59.02741602015059}, {"position"=140.76002941176475, "velocity"=71.99411764705881, "acceleration"=1.1764705882342241, "jerk"=-58.823529411853315, "heading"=58.82875310063778}, {"position"=141.48000000000005, "velocity"=72.0, "acceleration"=0.5882352941185331, "jerk"=-58.8235294115691, "heading"=58.62321433998458}, {"position"=142.20000000000005, "velocity"=72.0, "acceleration"=0.0, "jerk"=-58.823529411853315, "heading"=58.41074384530142}, {"position"=142.92000000000004, "velocity"=72.0, "acceleration"=0.0, "jerk"=0.0, "heading"=58.191274633471544}, {"position"=143.64000000000004, "velocity"=72.0, "acceleration"=0.0, "jerk"=0.0, "heading"=57.96473050504769}, {"position"=144.36000000000004, "velocity"=72.0, "acceleration"=0.0, "jerk"=0.0, "heading"=57.73103528357078}, {"position"=145.08000000000004, "velocity"=72.0, "acceleration"=0.0, "jerk"=0.0, "heading"=57.49010846075382}, {"position"=145.80000000000004, "velocity"=72.0, "acceleration"=0.0, "jerk"=0.0, "heading"=57.241872750728334}, {"position"=146.52000000000004, "velocity"=72.0, "acceleration"=0.0, "jerk"=0.0, "heading"=56.98624457558096}, {"position"=147.24000000000004, "velocity"=72.0, "acceleration"=0.0, "jerk"=0.0, "heading"=56.723145160895776}, {"position"=147.96000000000004, "velocity"=72.0, "acceleration"=0.0, "jerk"=0.0, "heading"=56.452489493580124}, {"position"=148.68000000000004, "velocity"=72.0, "acceleration"=0.0, "jerk"=0.0, "heading"=56.174196722878186}, {"position"=149.40000000000003, "velocity"=72.0, "acceleration"=0.0, "jerk"=0.0, "heading"=55.8881824483932}, {"position"=150.12000000000003, "velocity"=72.0, "acceleration"=0.0, "jerk"=0.0, "heading"=55.59436295853679}, {"position"=150.84000000000003, "velocity"=72.0, "acceleration"=0.0, "jerk"=0.0, "heading"=55.29265693174821}, {"position"=151.56000000000003, "velocity"=72.0, "acceleration"=0.0, "jerk"=0.0, "heading"=54.98297684165404}, {"position"=152.28000000000003, "velocity"=72.0, "acceleration"=0.0, "jerk"=0.0, "heading"=54.66524731814555}, {"position"=153.00000000000003, "velocity"=72.0, "acceleration"=0.0, "jerk"=0.0, "heading"=54.33937594181852}, {"position"=153.72000000000003, "velocity"=72.0, "acceleration"=0.0, "jerk"=0.0, "heading"=54.00529597341108}, {"position"=154.44000000000003, "velocity"=72.0, "acceleration"=0.0, "jerk"=0.0, "heading"=53.662910666936384}, {"position"=155.16000000000003, "velocity"=72.0, "acceleration"=0.0, "jerk"=0.0, "heading"=53.3121590026958}, {"position"=155.88000000000002, "velocity"=72.0, "acceleration"=0.0, "jerk"=0.0, "heading"=52.95295369091313}, {"position"=156.60000000000002, "velocity"=72.0, "acceleration"=0.0, "jerk"=0.0, "heading"=52.58522763729206}, {"position"=157.32000000000002, "velocity"=72.0, "acceleration"=0.0, "jerk"=0.0, "heading"=52.20891064053331}, {"position"=158.04000000000002, "velocity"=72.0, "acceleration"=0.0, "jerk"=0.0, "heading"=51.823928422933726}, {"position"=158.76000000000002, "velocity"=72.0, "acceleration"=0.0, "jerk"=0.0, "heading"=51.43022984629129}, {"position"=159.48000000000002, "velocity"=72.0, "acceleration"=0.0, "jerk"=0.0, "heading"=51.02773940525069}, {"position"=160.20000000000002, "velocity"=72.0, "acceleration"=0.0, "jerk"=0.0, "heading"=50.61641559765269}, {"position"=160.92000000000002, "velocity"=72.0, "acceleration"=0.0, "jerk"=0.0, "heading"=50.19620415060561}, {"position"=161.64000000000001, "velocity"=72.0, "acceleration"=0.0, "jerk"=0.0, "heading"=49.767055721767235}, {"position"=162.36, "velocity"=72.0, "acceleration"=0.0, "jerk"=0.0, "heading"=49.32894305188409}, {"position"=163.08, "velocity"=72.0, "acceleration"=0.0, "jerk"=0.0, "heading"=48.88182139877372}, {"position"=163.8, "velocity"=72.0, "acceleration"=0.0, "jerk"=0.0, "heading"=48.425675152317766}, {"position"=164.52, "velocity"=72.0, "acceleration"=0.0, "jerk"=0.0, "heading"=47.960489988110744}, {"position"=165.24, "velocity"=72.0, "acceleration"=0.0, "jerk"=0.0, "heading"=47.486244272025075}, {"position"=165.96, "velocity"=72.0, "acceleration"=0.0, "jerk"=0.0, "heading"=47.00295300381751}, {"position"=166.68, "velocity"=72.0, "acceleration"=0.0, "jerk"=0.0, "heading"=46.51062159055836}, {"position"=167.4, "velocity"=72.0, "acceleration"=0.0, "jerk"=0.0, "heading"=46.00926507826145}, {"position"=168.12, "velocity"=72.0, "acceleration"=0.0, "jerk"=0.0, "heading"=45.498924110532265}, {"position"=168.84, "velocity"=72.0, "acceleration"=0.0, "jerk"=0.0, "heading"=44.97963539454311}, {"position"=169.56, "velocity"=72.0, "acceleration"=0.0, "jerk"=0.0, "heading"=44.451452497104384}, {"position"=170.28, "velocity"=72.0, "acceleration"=0.0, "jerk"=0.0, "heading"=43.914448634994834}, {"position"=171.0, "velocity"=72.0, "acceleration"=0.0, "jerk"=0.0, "heading"=43.36869876767208}, {"position"=171.72, "velocity"=72.0, "acceleration"=0.0, "jerk"=0.0, "heading"=42.81429739880594}, {"position"=172.44, "velocity"=72.0, "acceleration"=0.0, "jerk"=0.0, "heading"=42.251356397480215}, {"position"=173.16, "velocity"=72.0, "acceleration"=0.0, "jerk"=0.0, "heading"=41.67999472789753}, {"position"=173.88, "velocity"=72.0, "acceleration"=0.0, "jerk"=0.0, "heading"=41.10035082283751}, {"position"=174.6, "velocity"=72.0, "acceleration"=0.0, "jerk"=0.0, "heading"=40.51257973836975}, {"position"=175.32, "velocity"=72.0, "acceleration"=0.0, "jerk"=0.0, "heading"=39.91684847399869}, {"position"=176.04, "velocity"=72.0, "acceleration"=0.0, "jerk"=0.0, "heading"=39.31334258704769}, {"position"=176.76, "velocity"=72.0, "acceleration"=0.0, "jerk"=0.0, "heading"=38.7022627005451}, {"position"=177.48, "velocity"=72.0, "acceleration"=0.0, "jerk"=0.0, "heading"=38.083825857157024}, {"position"=178.2, "velocity"=72.0, "acceleration"=0.0, "jerk"=0.0, "heading"=37.45826724146076}, {"position"=178.92, "velocity"=72.0, "acceleration"=0.0, "jerk"=0.0, "heading"=36.82583288981042}, {"position"=179.64, "velocity"=72.0, "acceleration"=0.0, "jerk"=0.0, "heading"=36.18678994469708}, {"position"=180.35999999999999, "velocity"=72.0, "acceleration"=0.0, "jerk"=0.0, "heading"=35.54142348582678}, {"position"=181.07999999999998, "velocity"=72.0, "acceleration"=0.0, "jerk"=0.0, "heading"=34.89002229615976}, {"position"=181.79999999999998, "velocity"=72.0, "acceleration"=0.0, "jerk"=0.0, "heading"=34.23290231067676}, {"position"=182.51999999999998, "velocity"=72.0, "acceleration"=0.0, "jerk"=0.0, "heading"=33.57039428579225}, {"position"=183.23999999999998, "velocity"=72.0, "acceleration"=0.0, "jerk"=0.0, "heading"=32.90282515257734}, {"position"=183.95999999999998, "velocity"=72.0, "acceleration"=0.0, "jerk"=0.0, "heading"=32.230558171726365}, {"position"=184.67999999999998, "velocity"=72.0, "acceleration"=0.0, "jerk"=0.0, "heading"=31.553958142486735}, {"position"=185.39999999999998, "velocity"=72.0, "acceleration"=0.0, "jerk"=0.0, "heading"=30.87338487221283}, {"position"=186.11999999999998, "velocity"=72.0, "acceleration"=0.0, "jerk"=0.0, "heading"=30.189249164675296}, {"position"=186.83999999999997, "velocity"=72.0, "acceleration"=0.0, "jerk"=0.0, "heading"=29.501927358393242}, {"position"=187.55999999999997, "velocity"=72.0, "acceleration"=0.0, "jerk"=0.0, "heading"=28.8118146643286}, {"position"=188.27999999999997, "velocity"=72.0, "acceleration"=0.0, "jerk"=0.0, "heading"=28.119354198013895}, {"position"=188.99999999999997, "velocity"=72.0, "acceleration"=0.0, "jerk"=0.0, "heading"=27.424916291244358}, {"position"=189.71999999999997, "velocity"=72.0, "acceleration"=0.0, "jerk"=0.0, "heading"=26.728952840958996}, {"position"=190.43999999999997, "velocity"=72.0, "acceleration"=0.0, "jerk"=0.0, "heading"=26.031866651472473}, {"position"=191.15999999999997, "velocity"=72.0, "acceleration"=0.0, "jerk"=0.0, "heading"=25.334072708234384}, {"position"=191.87999999999997, "velocity"=72.0, "acceleration"=0.0, "jerk"=0.0, "heading"=24.636021556146396}, {"position"=192.59999999999997, "velocity"=72.0, "acceleration"=0.0, "jerk"=0.0, "heading"=23.938080373815527}, {"position"=193.31999999999996, "velocity"=72.0, "acceleration"=0.0, "jerk"=0.0, "heading"=23.24073741189025}, {"position"=194.03999999999996, "velocity"=72.0, "acceleration"=0.0, "jerk"=0.0, "heading"=22.54431697414893}, {"position"=194.75999999999996, "velocity"=72.0, "acceleration"=0.0, "jerk"=0.0, "heading"=21.849319260906412}, {"position"=195.47999999999996, "velocity"=72.0, "acceleration"=0.0, "jerk"=0.0, "heading"=21.156040230089108}, {"position"=196.19999999999996, "velocity"=72.0, "acceleration"=0.0, "jerk"=0.0, "heading"=20.464976813329844}, {"position"=196.91999999999996, "velocity"=72.0, "acceleration"=0.0, "jerk"=0.0, "heading"=19.77640093707042}, {"position"=197.63999999999996, "velocity"=72.0, "acceleration"=0.0, "jerk"=0.0, "heading"=19.09078341794313}, {"position"=198.35999999999996, "velocity"=72.0, "acceleration"=0.0, "jerk"=0.0, "heading"=18.408396017236825}, {"position"=199.07999999999996, "velocity"=72.0, "acceleration"=0.0, "jerk"=0.0, "heading"=17.729639257609474}, {"position"=199.79999999999995, "velocity"=72.0, "acceleration"=0.0, "jerk"=0.0, "heading"=17.05482666802146}, {"position"=200.51999999999995, "velocity"=72.0, "acceleration"=0.0, "jerk"=0.0, "heading"=16.384239816139416}, {"position"=201.23999999999995, "velocity"=72.0, "acceleration"=0.0, "jerk"=0.0, "heading"=15.718278037263369}, {"position"=201.95999999999995, "velocity"=72.0, "acceleration"=0.0, "jerk"=0.0, "heading"=15.057129834341575}, {"position"=202.67999999999995, "velocity"=72.0, "acceleration"=0.0, "jerk"=0.0, "heading"=14.401094567436195}, {"position"=203.39999999999995, "velocity"=72.0, "acceleration"=0.0, "jerk"=0.0, "heading"=13.75048617704502}, {"position"=204.11999999999995, "velocity"=72.0, "acceleration"=0.0, "jerk"=0.0, "heading"=13.105468818025589}, {"position"=204.83999999999995, "velocity"=72.0, "acceleration"=0.0, "jerk"=0.0, "heading"=12.466270307758526}, {"position"=205.55999999999995, "velocity"=72.0, "acceleration"=0.0, "jerk"=0.0, "heading"=11.83317926731963}, {"position"=206.27999999999994, "velocity"=72.0, "acceleration"=0.0, "jerk"=0.0, "heading"=11.206323761876378}, {"position"=206.99999999999994, "velocity"=72.0, "acceleration"=0.0, "jerk"=0.0, "heading"=10.585870854147643}, {"position"=207.71999999999994, "velocity"=72.0, "acceleration"=0.0, "jerk"=0.0, "heading"=9.971984301316105}, {"position"=208.43999999999994, "velocity"=72.0, "acceleration"=0.0, "jerk"=0.0, "heading"=9.364837203968845}, {"position"=209.15999999999994, "velocity"=72.0, "acceleration"=0.0, "jerk"=0.0, "heading"=8.764573787885586}, {"position"=209.87999999999994, "velocity"=72.0, "acceleration"=0.0, "jerk"=0.0, "heading"=8.171269738717564}, {"position"=210.59999999999994, "velocity"=72.0, "acceleration"=0.0, "jerk"=0.0, "heading"=7.585027919971222}, {"position"=211.31999999999994, "velocity"=72.0, "acceleration"=0.0, "jerk"=0.0, "heading"=7.005937004518697}, {"position"=212.03999999999994, "velocity"=72.0, "acceleration"=0.0, "jerk"=0.0, "heading"=6.43407192082134}, {"position"=212.75999999999993, "velocity"=72.0, "acceleration"=0.0, "jerk"=0.0, "heading"=5.869494333123817}, {"position"=213.47999999999993, "velocity"=72.0, "acceleration"=0.0, "jerk"=0.0, "heading"=5.31225315022276}, {"position"=214.19999999999993, "velocity"=72.0, "acceleration"=0.0, "jerk"=0.0, "heading"=4.762385057601569}, {"position"=214.91999999999993, "velocity"=72.0, "acceleration"=0.0, "jerk"=0.0, "heading"=4.219915067949077}, {"position"=215.63999999999993, "velocity"=72.0, "acceleration"=0.0, "jerk"=0.0, "heading"=3.6848570853418394}, {"position"=216.35999999999993, "velocity"=72.0, "acceleration"=0.0, "jerk"=0.0, "heading"=3.15721447865805}, {"position"=217.07999999999993, "velocity"=72.0, "acceleration"=0.0, "jerk"=0.0, "heading"=2.636980660100461}, {"position"=217.79999999999993, "velocity"=72.0, "acceleration"=0.0, "jerk"=0.0, "heading"=2.1241396650258997}, {"position"=218.51999999999992, "velocity"=72.0, "acceleration"=0.0, "jerk"=0.0, "heading"=1.618666729610987}, {"position"=219.23999999999992, "velocity"=72.0, "acceleration"=0.0, "jerk"=0.0, "heading"=1.1205288632149972}, {"position"=219.95999999999992, "velocity"=72.0, "acceleration"=0.0, "jerk"=0.0, "heading"=0.6296854126303496}, {"position"=220.67999999999992, "velocity"=72.0, "acceleration"=0.0, "jerk"=0.0, "heading"=0.14608861573723728}, {"position"=221.39999999999992, "velocity"=72.0, "acceleration"=0.0, "jerk"=0.0, "heading"=359.8277826692572}, {"position"=222.11999999999992, "velocity"=72.0, "acceleration"=0.0, "jerk"=0.0, "heading"=359.4648535883929}, {"position"=222.83999999999992, "velocity"=72.0, "acceleration"=0.0, "jerk"=0.0, "heading"=359.09466236597694}, {"position"=223.55999999999992, "velocity"=72.0, "acceleration"=0.0, "jerk"=0.0, "heading"=358.7170518068175}, {"position"=224.27999999999992, "velocity"=72.0, "acceleration"=0.0, "jerk"=0.0, "heading"=358.33182788568945}, {"position"=224.99999999999991, "velocity"=72.0, "acceleration"=0.0, "jerk"=0.0, "heading"=357.93879262657174}, {"position"=225.7199999999999, "velocity"=72.0, "acceleration"=0.0, "jerk"=0.0, "heading"=357.53774421338426}, {"position"=226.4399999999999, "velocity"=72.0, "acceleration"=0.0, "jerk"=0.0, "heading"=357.12847712681753}, {"position"=227.1599999999999, "velocity"=72.0, "acceleration"=0.0, "jerk"=0.0, "heading"=356.71078230983005}, {"position"=227.8799999999999, "velocity"=72.0, "acceleration"=0.0, "jerk"=0.0, "heading"=356.2844473645489}, {"position"=228.5999999999999, "velocity"=72.0, "acceleration"=0.0, "jerk"=0.0, "heading"=355.849256783469}, {"position"=229.3199999999999, "velocity"=72.0, "acceleration"=0.0, "jerk"=0.0, "heading"=355.40499221800604}, {"position"=230.0399999999999, "velocity"=72.0, "acceleration"=0.0, "jerk"=0.0, "heading"=354.9514327876068}, {"position"=230.7599999999999, "velocity"=72.0, "acceleration"=0.0, "jerk"=0.0, "heading"=354.48835543276255}, {"position"=231.4799999999999, "velocity"=72.0, "acceleration"=0.0, "jerk"=0.0, "heading"=354.015535315402}, {"position"=232.1999999999999, "velocity"=72.0, "acceleration"=0.0, "jerk"=0.0, "heading"=353.53271733266087}, {"position"=232.9199999999999, "velocity"=72.0, "acceleration"=0.0, "jerk"=0.0, "heading"=353.03968265986583}, {"position"=233.6399999999999, "velocity"=72.0, "acceleration"=0.0, "jerk"=0.0, "heading"=352.5362173129394}, {"position"=234.3599999999999, "velocity"=72.0, "acceleration"=0.0, "jerk"=0.0, "heading"=352.02204329715573}, {"position"=235.0799999999999, "velocity"=72.0, "acceleration"=0.0, "jerk"=0.0, "heading"=351.49696474764124}, {"position"=235.7999999999999, "velocity"=72.0, "acceleration"=0.0, "jerk"=0.0, "heading"=350.96071959819545}, {"position"=236.5199999999999, "velocity"=72.0, "acceleration"=0.0, "jerk"=0.0, "heading"=350.4131006027368}, {"position"=237.2399999999999, "velocity"=72.0, "acceleration"=0.0, "jerk"=0.0, "heading"=349.8538382014103}, {"position"=237.9599999999999, "velocity"=72.0, "acceleration"=0.0, "jerk"=0.0, "heading"=349.2827468492259}, {"position"=238.6799999999999, "velocity"=72.0, "acceleration"=0.0, "jerk"=0.0, "heading"=348.69957980356105}, {"position"=239.3999999999999, "velocity"=72.0, "acceleration"=0.0, "jerk"=0.0, "heading"=348.10410705007126}, {"position"=240.1199999999999, "velocity"=72.0, "acceleration"=0.0, "jerk"=0.0, "heading"=347.4961404042255}, {"position"=240.8399999999999, "velocity"=72.0, "acceleration"=0.0, "jerk"=0.0, "heading"=346.87547263645445}, {"position"=241.5599999999999, "velocity"=72.0, "acceleration"=0.0, "jerk"=0.0, "heading"=346.2419075046829}, {"position"=242.2799999999999, "velocity"=72.0, "acceleration"=0.0, "jerk"=0.0, "heading"=345.5952614922891}, {"position"=242.9999999999999, "velocity"=72.0, "acceleration"=0.0, "jerk"=0.0, "heading"=344.935365651339}, {"position"=243.71999999999989, "velocity"=72.0, "acceleration"=0.0, "jerk"=0.0, "heading"=344.2620675468098}, {"position"=244.43999999999988, "velocity"=72.0, "acceleration"=0.0, "jerk"=0.0, "heading"=343.575233295516}, {"position"=245.15999999999988, "velocity"=72.0, "acceleration"=0.0, "jerk"=0.0, "heading"=342.87474969121354}, {"position"=245.87999999999988, "velocity"=72.0, "acceleration"=0.0, "jerk"=0.0, "heading"=342.16052640490784}, {"position"=246.59999999999988, "velocity"=72.0, "acceleration"=0.0, "jerk"=0.0, "heading"=341.43248206997083}, {"position"=247.31999999999988, "velocity"=72.0, "acceleration"=0.0, "jerk"=0.0, "heading"=340.6905614599298}, {"position"=248.03999999999988, "velocity"=72.0, "acceleration"=0.0, "jerk"=0.0, "heading"=339.93478326841307}, {"position"=248.75999999999988, "velocity"=72.0, "acceleration"=0.0, "jerk"=0.0, "heading"=339.1651350290684}, {"position"=249.47999999999988, "velocity"=72.0, "acceleration"=0.0, "jerk"=0.0, "heading"=338.3816789738869}, {"position"=250.19999999999987, "velocity"=72.0, "acceleration"=0.0, "jerk"=0.0, "heading"=337.5845001034723}, {"position"=250.91999999999987, "velocity"=72.0, "acceleration"=0.0, "jerk"=0.0, "heading"=336.7737284965488}, {"position"=251.63999999999987, "velocity"=72.0, "acceleration"=0.0, "jerk"=0.0, "heading"=335.94951132318914}, {"position"=252.35999999999987, "velocity"=72.0, "acceleration"=0.0, "jerk"=0.0, "heading"=335.112088819133}, {"position"=253.07999999999987, "velocity"=72.0, "acceleration"=0.0, "jerk"=0.0, "heading"=334.2616979005428}, {"position"=253.79999999999987, "velocity"=72.0, "acceleration"=0.0, "jerk"=0.0, "heading"=333.3986304515005}, {"position"=254.51999999999987, "velocity"=72.0, "acceleration"=0.0, "jerk"=0.0, "heading"=332.5232581495264}, {"position"=255.23999999999987, "velocity"=72.0, "acceleration"=0.0, "jerk"=0.0, "heading"=331.6359794566513}, {"position"=255.95999999999987, "velocity"=72.0, "acceleration"=0.0, "jerk"=0.0, "heading"=330.7372450462164}, {"position"=256.6799999999999, "velocity"=72.0, "acceleration"=0.0, "jerk"=0.0, "heading"=329.8275581349173}, {"position"=257.3999999999999, "velocity"=72.0, "acceleration"=0.0, "jerk"=0.0, "heading"=328.9074743383309}, {"position"=258.11999999999995, "velocity"=72.0, "acceleration"=0.0, "jerk"=0.0, "heading"=327.97760101633475}, {"position"=258.84, "velocity"=72.0, "acceleration"=0.0, "jerk"=0.0, "heading"=327.038596082075}, {"position"=259.56, "velocity"=72.0, "acceleration"=0.0, "jerk"=0.0, "heading"=326.09116625673795}, {"position"=260.28000000000003, "velocity"=72.0, "acceleration"=0.0, "jerk"=0.0, "heading"=325.13606476218604}, {"position"=261.00000000000006, "velocity"=72.0, "acceleration"=0.0, "jerk"=0.0, "heading"=324.1740884543122}, {"position"=261.7200000000001, "velocity"=72.0, "acceleration"=0.0, "jerk"=0.0, "heading"=323.20605712446866}, {"position"=262.4400000000001, "velocity"=72.0, "acceleration"=0.0, "jerk"=0.0, "heading"=322.23285924189577}, {"position"=263.16000000000014, "velocity"=72.0, "acceleration"=0.0, "jerk"=0.0, "heading"=321.2554030865098}, {"position"=263.88000000000017, "velocity"=72.0, "acceleration"=0.0, "jerk"=0.0, "heading"=320.2746141632579}, {"position"=264.6000000000002, "velocity"=72.0, "acceleration"=0.0, "jerk"=0.0, "heading"=319.29144178208156}, {"position"=265.3200000000002, "velocity"=72.0, "acceleration"=0.0, "jerk"=0.0, "heading"=318.3068723390094}, {"position"=266.04000000000025, "velocity"=72.0, "acceleration"=0.0, "jerk"=0.0, "heading"=317.3218759034037}, {"position"=266.7600000000003, "velocity"=72.0, "acceleration"=0.0, "jerk"=0.0, "heading"=316.33744638729615}, {"position"=267.4800000000003, "velocity"=72.0, "acceleration"=0.0, "jerk"=0.0, "heading"=315.35457311156046}, {"position"=268.20000000000033, "velocity"=72.0, "acceleration"=0.0, "jerk"=0.0, "heading"=314.3742285191228}, {"position"=268.92000000000036, "velocity"=72.0, "acceleration"=0.0, "jerk"=0.0, "heading"=313.3973903081687}, {"position"=269.6400000000004, "velocity"=72.0, "acceleration"=0.0, "jerk"=0.0, "heading"=312.424996516643}, {"position"=270.3600000000004, "velocity"=72.0, "acceleration"=0.0, "jerk"=0.0, "heading"=311.4579820085233}, {"position"=271.08000000000044, "velocity"=72.0, "acceleration"=0.0, "jerk"=0.0, "heading"=310.49723488949087}, {"position"=271.80000000000047, "velocity"=72.0, "acceleration"=0.0, "jerk"=0.0, "heading"=309.5436227425424}, {"position"=272.5200000000005, "velocity"=72.0, "acceleration"=0.0, "jerk"=0.0, "heading"=308.597966676722}, {"position"=273.2400000000005, "velocity"=72.0, "acceleration"=0.0, "jerk"=0.0, "heading"=307.6610501714979}, {"position"=273.96000000000055, "velocity"=72.0, "acceleration"=0.0, "jerk"=0.0, "heading"=306.73361209819114}, {"position"=274.6800000000006, "velocity"=72.0, "acceleration"=0.0, "jerk"=0.0, "heading"=305.81634021610245}, {"position"=275.4000000000006, "velocity"=72.0, "acceleration"=0.0, "jerk"=0.0, "heading"=304.90988006904456}, {"position"=276.12000000000063, "velocity"=72.0, "acceleration"=0.0, "jerk"=0.0, "heading"=304.0148168458594}, {"position"=276.84000000000066, "velocity"=72.0, "acceleration"=0.0, "jerk"=0.0, "heading"=303.13169549130475}, {"position"=277.5600000000007, "velocity"=72.0, "acceleration"=0.0, "jerk"=0.0, "heading"=302.26099730482406}, {"position"=278.2800000000007, "velocity"=72.0, "acceleration"=0.0, "jerk"=0.0, "heading"=301.4031622246539}, {"position"=279.00000000000074, "velocity"=72.0, "acceleration"=0.0, "jerk"=0.0, "heading"=300.55857197058}, {"position"=279.72000000000077, "velocity"=72.0, "acceleration"=0.0, "jerk"=0.0, "heading"=299.7275590703089}, {"position"=280.4400000000008, "velocity"=72.0, "acceleration"=0.0, "jerk"=0.0, "heading"=298.91041514787196}, {"position"=281.1600000000008, "velocity"=72.0, "acceleration"=0.0, "jerk"=0.0, "heading"=298.1073684085312}, {"position"=281.88000000000085, "velocity"=72.0, "acceleration"=0.0, "jerk"=0.0, "heading"=297.31862157642985}, {"position"=282.6000000000009, "velocity"=72.0, "acceleration"=0.0, "jerk"=0.0, "heading"=296.5443192880639}, {"position"=283.3200000000009, "velocity"=72.0, "acceleration"=0.0, "jerk"=0.0, "heading"=295.7845665770592}, {"position"=284.04000000000093, "velocity"=72.0, "acceleration"=0.0, "jerk"=0.0, "heading"=295.0394433568115}, {"position"=284.76000000000096, "velocity"=72.0, "acceleration"=0.0, "jerk"=0.0, "heading"=294.30897952077703}, {"position"=285.480000000001, "velocity"=72.0, "acceleration"=0.0, "jerk"=0.0, "heading"=293.59317299852836}, {"position"=286.200000000001, "velocity"=72.0, "acceleration"=0.0, "jerk"=0.0, "heading"=292.8919948905544}, {"position"=286.92000000000104, "velocity"=72.0, "acceleration"=0.0, "jerk"=0.0, "heading"=292.2053952701814}, {"position"=287.64000000000107, "velocity"=72.0, "acceleration"=0.0, "jerk"=0.0, "heading"=291.5332849029608}, {"position"=288.3600000000011, "velocity"=72.0, "acceleration"=0.0, "jerk"=0.0, "heading"=290.8755552287482}, {"position"=289.0800000000011, "velocity"=72.0, "acceleration"=0.0, "jerk"=0.0, "heading"=290.23207861143834}, {"position"=289.80000000000115, "velocity"=72.0, "acceleration"=0.0, "jerk"=0.0, "heading"=289.60270852380256}, {"position"=290.5200000000012, "velocity"=72.0, "acceleration"=0.0, "jerk"=0.0, "heading"=288.987281664332}, {"position"=291.2400000000012, "velocity"=72.0, "acceleration"=0.0, "jerk"=0.0, "heading"=288.3856199666264}, {"position"=291.96000000000123, "velocity"=72.0, "acceleration"=0.0, "jerk"=0.0, "heading"=287.79753249585394}, {"position"=292.68000000000126, "velocity"=72.0, "acceleration"=0.0, "jerk"=0.0, "heading"=287.2228172289517}, {"position"=293.4000000000013, "velocity"=72.0, "acceleration"=0.0, "jerk"=0.0, "heading"=286.66126271710476}, {"position"=294.1200000000013, "velocity"=72.0, "acceleration"=0.0, "jerk"=0.0, "heading"=286.11264963064014}, {"position"=294.84000000000134, "velocity"=72.0, "acceleration"=0.0, "jerk"=0.0, "heading"=285.57675218782055}, {"position"=295.56000000000137, "velocity"=72.0, "acceleration"=0.0, "jerk"=0.0, "heading"=285.05333947012645}, {"position"=296.2800000000014, "velocity"=72.0, "acceleration"=0.0, "jerk"=0.0, "heading"=284.5421766275192}, {"position"=297.0000000000014, "velocity"=72.0, "acceleration"=0.0, "jerk"=0.0, "heading"=284.04302597787506}, {"position"=297.72000000000145, "velocity"=72.0, "acceleration"=0.0, "jerk"=0.0, "heading"=283.5556480053136}, {"position"=298.4400000000015, "velocity"=72.0, "acceleration"=0.0, "jerk"=0.0, "heading"=283.07981074612997}, {"position"=299.1600000000015, "velocity"=72.0, "acceleration"=0.0, "jerk"=0.0, "heading"=282.61526646843146}, {"position"=299.88000000000153, "velocity"=72.0, "acceleration"=0.0, "jerk"=0.0, "heading"=282.161774504175}, {"position"=300.60000000000156, "velocity"=72.0, "acceleration"=0.0, "jerk"=0.0, "heading"=281.71909772914074}, {"position"=301.3200000000016, "velocity"=72.0, "acceleration"=0.0, "jerk"=0.0, "heading"=281.2870080661241}, {"position"=302.0400000000016, "velocity"=72.0, "acceleration"=0.0, "jerk"=0.0, "heading"=280.86526069319876}, {"position"=302.76000000000164, "velocity"=72.0, "acceleration"=0.0, "jerk"=0.0, "heading"=280.45362760401355}, {"position"=303.48000000000167, "velocity"=72.0, "acceleration"=0.0, "jerk"=0.0, "heading"=280.05188609921316}, {"position"=304.2000000000017, "velocity"=72.0, "acceleration"=0.0, "jerk"=0.0, "heading"=279.6598009868634}, {"position"=304.9200000000017, "velocity"=72.0, "acceleration"=0.0, "jerk"=0.0, "heading"=279.2771639643657}, {"position"=305.64000000000175, "velocity"=72.0, "acceleration"=0.0, "jerk"=0.0, "heading"=278.9037458491646}, {"position"=306.3600000000018, "velocity"=72.0, "acceleration"=0.0, "jerk"=0.0, "heading"=278.53934356113734}, {"position"=307.0800000000018, "velocity"=72.0, "acceleration"=0.0, "jerk"=0.0, "heading"=278.1837394357979}, {"position"=307.80000000000183, "velocity"=72.0, "acceleration"=0.0, "jerk"=0.0, "heading"=277.8367388857313}, {"position"=308.52000000000186, "velocity"=72.0, "acceleration"=0.0, "jerk"=0.0, "heading"=277.4981315006348}, {"position"=309.2400000000019, "velocity"=72.0, "acceleration"=0.0, "jerk"=0.0, "heading"=277.1677334984439}, {"position"=309.9600000000019, "velocity"=72.0, "acceleration"=0.0, "jerk"=0.0, "heading"=276.8453452726322}, {"position"=310.68000000000194, "velocity"=72.0, "acceleration"=0.0, "jerk"=0.0, "heading"=276.5307834904454}, {"position"=311.40000000000197, "velocity"=72.0, "acceleration"=0.0, "jerk"=0.0, "heading"=276.2238709422801}, {"position"=312.120000000002, "velocity"=72.0, "acceleration"=0.0, "jerk"=0.0, "heading"=275.92442494953866}, {"position"=312.840000000002, "velocity"=72.0, "acceleration"=0.0, "jerk"=0.0, "heading"=275.63227552213914}, {"position"=313.56000000000205, "velocity"=72.0, "acceleration"=0.0, "jerk"=0.0, "heading"=275.3472597649053}, {"position"=314.2800000000021, "velocity"=72.0, "acceleration"=0.0, "jerk"=0.0, "heading"=275.06920944903135}, {"position"=315.0000000000021, "velocity"=72.0, "acceleration"=0.0, "jerk"=0.0, "heading"=274.7979667641207}, {"position"=315.72000000000213, "velocity"=72.0, "acceleration"=0.0, "jerk"=0.0, "heading"=274.5333789111209}, {"position"=316.44000000000216, "velocity"=72.0, "acceleration"=0.0, "jerk"=0.0, "heading"=274.2752993969795}, {"position"=317.1600000000022, "velocity"=72.0, "acceleration"=0.0, "jerk"=0.0, "heading"=274.02357937814594}, {"position"=317.8800000000022, "velocity"=72.0, "acceleration"=0.0, "jerk"=0.0, "heading"=273.7780781726711}, {"position"=318.60000000000224, "velocity"=72.0, "acceleration"=0.0, "jerk"=0.0, "heading"=273.53865919532046}, {"position"=319.32000000000227, "velocity"=72.0, "acceleration"=0.0, "jerk"=0.0, "heading"=273.3051898816098}, {"position"=320.0400000000023, "velocity"=72.0, "acceleration"=0.0, "jerk"=0.0, "heading"=273.07754160915556}, {"position"=320.7600000000023, "velocity"=72.0, "acceleration"=0.0, "jerk"=0.0, "heading"=272.8555899320782}, {"position"=321.48000000000235, "velocity"=72.0, "acceleration"=0.0, "jerk"=0.0, "heading"=272.63921435109694}, {"position"=322.2000000000024, "velocity"=72.0, "acceleration"=0.0, "jerk"=0.0, "heading"=272.42829644947125}, {"position"=322.9200000000024, "velocity"=72.0, "acceleration"=0.0, "jerk"=0.0, "heading"=272.22272258890786}, {"position"=323.64000000000243, "velocity"=72.0, "acceleration"=0.0, "jerk"=0.0, "heading"=272.0223826566521}, {"position"=324.36000000000246, "velocity"=72.0, "acceleration"=0.0, "jerk"=0.0, "heading"=271.8271699814326}, {"position"=325.0800000000025, "velocity"=72.0, "acceleration"=0.0, "jerk"=0.0, "heading"=271.63698124978595}, {"position"=325.8000000000025, "velocity"=72.0, "acceleration"=0.0, "jerk"=0.0, "heading"=271.4517164230191}, {"position"=326.52000000000254, "velocity"=72.0, "acceleration"=0.0, "jerk"=0.0, "heading"=271.2712786550298}, {"position"=327.24000000000257, "velocity"=72.0, "acceleration"=0.0, "jerk"=0.0, "heading"=271.09557421117904}, {"position"=327.9600000000026, "velocity"=72.0, "acceleration"=0.0, "jerk"=0.0, "heading"=270.9245123883809}, {"position"=328.6800000000026, "velocity"=72.0, "acceleration"=0.0, "jerk"=0.0, "heading"=270.7580059125007}, {"position"=329.40000000000265, "velocity"=72.0, "acceleration"=0.0, "jerk"=0.0, "heading"=270.59596985280666}, {"position"=330.1200000000027, "velocity"=72.0, "acceleration"=0.0, "jerk"=0.0, "heading"=270.43832175855033}, {"position"=330.8400000000027, "velocity"=72.0, "acceleration"=0.0, "jerk"=0.0, "heading"=270.2849822663125}, {"position"=331.56000000000273, "velocity"=72.0, "acceleration"=0.0, "jerk"=0.0, "heading"=270.1358746685782}, {"position"=332.28000000000276, "velocity"=72.0, "acceleration"=0.0, "jerk"=0.0, "heading"=270.0}, {"position"=333.0000000000028, "velocity"=72.0, "acceleration"=0.0, "jerk"=0.0, "heading"=270.0}, {"position"=333.7200000000028, "velocity"=72.0, "acceleration"=0.0, "jerk"=0.0, "heading"=270.0}, {"position"=334.44000000000284, "velocity"=72.0, "acceleration"=0.0, "jerk"=0.0, "heading"=270.0}, {"position"=335.16000000000287, "velocity"=72.0, "acceleration"=0.0, "jerk"=0.0, "heading"=270.0}, {"position"=335.8800000000029, "velocity"=72.0, "acceleration"=0.0, "jerk"=0.0, "heading"=270.0}, {"position"=336.6000000000029, "velocity"=72.0, "acceleration"=0.0, "jerk"=0.0, "heading"=270.0}, {"position"=337.32000000000295, "velocity"=72.0, "acceleration"=0.0, "jerk"=0.0, "heading"=270.0}, {"position"=338.040000000003, "velocity"=72.0, "acceleration"=0.0, "jerk"=0.0, "heading"=270.0}, {"position"=338.760000000003, "velocity"=72.0, "acceleration"=0.0, "jerk"=0.0, "heading"=270.0}, {"position"=339.48000000000303, "velocity"=72.0, "acceleration"=0.0, "jerk"=0.0, "heading"=270.0}, {"position"=340.20000000000306, "velocity"=72.0, "acceleration"=0.0, "jerk"=0.0, "heading"=270.0}, {"position"=340.9200000000031, "velocity"=72.0, "acceleration"=0.0, "jerk"=0.0, "heading"=270.0}, {"position"=341.6400000000031, "velocity"=72.0, "acceleration"=0.0, "jerk"=0.0, "heading"=270.0}, {"position"=342.36000000000314, "velocity"=72.0, "acceleration"=0.0, "jerk"=0.0, "heading"=270.0}, {"position"=343.08000000000317, "velocity"=72.0, "acceleration"=0.0, "jerk"=0.0, "heading"=270.0}, {"position"=343.8000000000032, "velocity"=72.0, "acceleration"=0.0, "jerk"=0.0, "heading"=270.0}, {"position"=344.5200000000032, "velocity"=72.0, "acceleration"=0.0, "jerk"=0.0, "heading"=270.0}, {"position"=345.24000000000325, "velocity"=72.0, "acceleration"=0.0, "jerk"=0.0, "heading"=270.0}, {"position"=345.9600000000033, "velocity"=72.0, "acceleration"=0.0, "jerk"=0.0, "heading"=270.0}, {"position"=346.6800000000033, "velocity"=72.0, "acceleration"=0.0, "jerk"=0.0, "heading"=270.0}, {"position"=347.40000000000333, "velocity"=72.0, "acceleration"=0.0, "jerk"=0.0, "heading"=270.0}, {"position"=348.12000000000336, "velocity"=72.0, "acceleration"=0.0, "jerk"=0.0, "heading"=270.0}, {"position"=348.8400000000034, "velocity"=72.0, "acceleration"=0.0, "jerk"=0.0, "heading"=270.0}, {"position"=349.5600000000034, "velocity"=72.0, "acceleration"=0.0, "jerk"=0.0, "heading"=270.0}, {"position"=350.28000000000344, "velocity"=72.0, "acceleration"=0.0, "jerk"=0.0, "heading"=270.0}, {"position"=351.00000000000347, "velocity"=72.0, "acceleration"=0.0, "jerk"=0.0, "heading"=270.0}, {"position"=351.7200000000035, "velocity"=72.0, "acceleration"=0.0, "jerk"=0.0, "heading"=270.0}, {"position"=352.4400000000035, "velocity"=72.0, "acceleration"=0.0, "jerk"=0.0, "heading"=270.0}, {"position"=353.16000000000355, "velocity"=72.0, "acceleration"=0.0, "jerk"=0.0, "heading"=270.0}, {"position"=353.8800000000036, "velocity"=72.0, "acceleration"=0.0, "jerk"=0.0, "heading"=270.0}, {"position"=354.6000000000036, "velocity"=72.0, "acceleration"=0.0, "jerk"=0.0, "heading"=270.0}, {"position"=355.32000000000363, "velocity"=72.0, "acceleration"=0.0, "jerk"=0.0, "heading"=270.0}, {"position"=356.04000000000366, "velocity"=72.0, "acceleration"=0.0, "jerk"=0.0, "heading"=270.0}, {"position"=356.7600000000037, "velocity"=72.0, "acceleration"=0.0, "jerk"=0.0, "heading"=270.0}, {"position"=357.4800000000037, "velocity"=72.0, "acceleration"=0.0, "jerk"=0.0, "heading"=270.0}, {"position"=358.20000000000374, "velocity"=72.0, "acceleration"=0.0, "jerk"=0.0, "heading"=270.0}, {"position"=358.92000000000377, "velocity"=72.0, "acceleration"=0.0, "jerk"=0.0, "heading"=270.0}, {"position"=359.63999360458337, "velocity"=71.99872091591678, "acceleration"=-0.12790840832224148, "jerk"=-12.790840832224148, "heading"=270.0}, {"position"=360.35994500655744, "velocity"=71.99155947889238, "acceleration"=-0.7161437024393535, "jerk"=-58.823529411711206, "heading"=270.0}, {"position"=361.0797953823965, "velocity"=71.97851568892682, "acceleration"=-1.3043789965564656, "jerk"=-58.823529411711206, "heading"=270.0}, {"position"=361.7994859085713, "velocity"=71.9595895460201, "acceleration"=-1.8926142906721566, "jerk"=-58.8235294115691, "heading"=270.0}, {"position"=362.51895776155226, "velocity"=71.93478105017216, "acceleration"=-2.480849584793532, "jerk"=-58.82352941213753, "heading"=270.0}, {"position"=363.23815211781005, "velocity"=71.90409020138306, "acceleration"=-3.069084878910644, "jerk"=-58.823529411711206, "heading"=270.0}, {"position"=363.95701015381525, "velocity"=71.86751699965279, "acceleration"=-3.657320173026335, "jerk"=-58.8235294115691, "heading"=270.0}, {"position"=364.6754730460384, "velocity"=71.82506144498134, "acceleration"=-4.245555467144868, "jerk"=-58.823529411853315, "heading"=270.0}, {"position"=365.3934819709502, "velocity"=71.77672353736872, "acceleration"=-4.83379076126198, "jerk"=-58.823529411711206, "heading"=270.0}, {"position"=366.1109781050211, "velocity"=71.7225032768149, "acceleration"=-5.422026055381934, "jerk"=-58.82352941199542, "heading"=270.0}, {"position"=366.8279026247218, "velocity"=71.66240066331993, "acceleration"=-6.010261349497625, "jerk"=-58.8235294115691, "heading"=270.0}, {"position"=367.5441967065228, "velocity"=71.59641569688378, "acceleration"=-6.598496643614737, "jerk"=-58.823529411711206, "heading"=270.0}, {"position"=368.25980152689476, "velocity"=71.52454837750643, "acceleration"=-7.186731937734692, "jerk"=-58.82352941199542, "heading"=270.0}, {"position"=368.97465826230825, "velocity"=71.44679870518793, "acceleration"=-7.774967231850383, "jerk"=-58.8235294115691, "heading"=270.0}, {"position"=369.68870808923384, "velocity"=71.36316667992824, "acceleration"=-8.363202525968916, "jerk"=-58.823529411853315, "heading"=270.0}, {"position"=370.4018921841421, "velocity"=71.27365230172738, "acceleration"=-8.951437820086028, "jerk"=-58.823529411711206, "heading"=270.0}, {"position"=371.1141517235037, "velocity"=71.17825557058534, "acceleration"=-9.539673114204561, "jerk"=-58.823529411853315, "heading"=270.0}, {"position"=371.82542788378913, "velocity"=71.07697648650212, "acceleration"=-10.127908408321673, "jerk"=-58.823529411711206, "heading"=270.0}, {"position"=372.53566184146905, "velocity"=70.96981504947773, "acceleration"=-10.716143702438785, "jerk"=-58.823529411711206, "heading"=270.0}, {"position"=373.244794773014, "velocity"=70.85677125951216, "acceleration"=-11.304378996557318, "jerk"=-58.823529411853315, "heading"=270.0}, {"position"=373.9527678548946, "velocity"=70.73784511660541, "acceleration"=-11.89261429067443, "jerk"=-58.823529411711206, "heading"=270.0}, {"position"=374.65952226358144, "velocity"=70.61303662075748, "acceleration"=-12.480849584792963, "jerk"=-58.823529411853315, "heading"=270.0}, {"position"=375.36499917554505, "velocity"=70.48234577196838, "acceleration"=-13.069084878910076, "jerk"=-58.823529411711206, "heading"=270.0}, {"position"=376.0691397672561, "velocity"=70.34577257023813, "acceleration"=-13.657320173025767, "jerk"=-58.8235294115691, "heading"=270.0}, {"position"=376.77188521518514, "velocity"=70.20331701556668, "acceleration"=-14.2455554671443, "jerk"=-58.823529411853315, "heading"=270.0}, {"position"=377.47317669580275, "velocity"=70.05497910795404, "acceleration"=-14.833790761264254, "jerk"=-58.82352941199542, "heading"=270.0}, {"position"=378.17295538557954, "velocity"=69.90075884740024, "acceleration"=-15.422026055379945, "jerk"=-58.8235294115691, "heading"=270.0}, {"position"=378.87116246098606, "velocity"=69.74065623390526, "acceleration"=-16.010261349498478, "jerk"=-58.823529411853315, "heading"=270.0}, {"position"=379.56773909849295, "velocity"=69.5746712674691, "acceleration"=-16.59849664361559, "jerk"=-58.823529411711206, "heading"=270.0}, {"position"=380.26262647457077, "velocity"=69.40280394809176, "acceleration"=-17.186731937734123, "jerk"=-58.823529411853315, "heading"=270.0}, {"position"=380.9557657656901, "velocity"=69.22505427577326, "acceleration"=-17.774967231849814, "jerk"=-58.8235294115691, "heading"=270.0}, {"position"=381.64709814832156, "velocity"=69.04142225051356, "acceleration"=-18.36320252596977, "jerk"=-58.82352941199542, "heading"=270.0}, {"position"=382.3365647989357, "velocity"=68.85190787231271, "acceleration"=-18.95143782008546, "jerk"=-58.8235294115691, "heading"=270.0}, {"position"=383.0241068940031, "velocity"=68.65651114117065, "acceleration"=-19.539673114205414, "jerk"=-58.82352941199542, "heading"=270.0}, {"position"=383.70967200541486, "velocity"=68.45651114117067, "acceleration"=-19.999999999998863, "jerk"=-46.03268857934495, "heading"=270.0}, {"position"=384.3932371168266, "velocity"=68.25651114117066, "acceleration"=-20.000000000000284, "jerk"=-1.4210854715202004e-10, "heading"=270.0}, {"position"=385.0748022282383, "velocity"=68.05651114117066, "acceleration"=-20.000000000000284, "jerk"=0.0, "heading"=270.0}, {"position"=385.75436733965, "velocity"=67.85651114117067, "acceleration"=-19.999999999998863, "jerk"=1.4210854715202004e-10, "heading"=270.0}, {"position"=386.4319324510617, "velocity"=67.65651114117065, "acceleration"=-20.000000000001705, "jerk"=-2.842170943040401e-10, "heading"=270.0}, {"position"=387.1074975624734, "velocity"=67.45651114117067, "acceleration"=-19.999999999998863, "jerk"=2.842170943040401e-10, "heading"=270.0}, {"position"=387.7810626738851, "velocity"=67.25651114117068, "acceleration"=-19.999999999998863, "jerk"=0.0, "heading"=270.0}, {"position"=388.45262778529684, "velocity"=67.05651114117066, "acceleration"=-20.000000000001705, "jerk"=-2.842170943040401e-10, "heading"=270.0}, {"position"=389.12219289670855, "velocity"=66.85651114117066, "acceleration"=-20.000000000000284, "jerk"=1.4210854715202004e-10, "heading"=270.0}, {"position"=389.78975800812026, "velocity"=66.65651114117067, "acceleration"=-19.999999999998863, "jerk"=1.4210854715202004e-10, "heading"=270.0}, {"position"=390.45532311953195, "velocity"=66.45651114117067, "acceleration"=-20.000000000000284, "jerk"=-1.4210854715202004e-10, "heading"=270.0}, {"position"=391.11888823094364, "velocity"=66.25651114117066, "acceleration"=-20.000000000000284, "jerk"=0.0, "heading"=270.0}, {"position"=391.7804533423554, "velocity"=66.05651114117066, "acceleration"=-20.000000000000284, "jerk"=0.0, "heading"=270.0}, {"position"=392.4400184537671, "velocity"=65.85651114117067, "acceleration"=-19.999999999998863, "jerk"=1.4210854715202004e-10, "heading"=270.0}, {"position"=393.0975835651788, "velocity"=65.65651114117067, "acceleration"=-20.000000000000284, "jerk"=-1.4210854715202004e-10, "heading"=270.0}, {"position"=393.7531486765905, "velocity"=65.45651114117067, "acceleration"=-20.000000000000284, "jerk"=0.0, "heading"=270.0}, {"position"=394.4067137880022, "velocity"=65.25651114117066, "acceleration"=-20.000000000000284, "jerk"=0.0, "heading"=270.0}, {"position"=395.0582788994139, "velocity"=65.05651114117066, "acceleration"=-20.000000000000284, "jerk"=0.0, "heading"=270.0}, {"position"=395.7078440108256, "velocity"=64.85651114117067, "acceleration"=-19.999999999998863, "jerk"=1.4210854715202004e-10, "heading"=270.0}, {"position"=396.35540912223735, "velocity"=64.65651114117067, "acceleration"=-20.000000000000284, "jerk"=-1.4210854715202004e-10, "heading"=270.0}, {"position"=397.00097423364906, "velocity"=64.45651114117067, "acceleration"=-20.000000000000284, "jerk"=0.0, "heading"=270.0}, {"position"=397.64453934506076, "velocity"=64.25651114117066, "acceleration"=-20.000000000000284, "jerk"=0.0, "heading"=270.0}, {"position"=398.28610445647246, "velocity"=64.05651114117066, "acceleration"=-20.000000000000284, "jerk"=0.0, "heading"=270.0}, {"position"=398.92566956788414, "velocity"=63.85651114117066, "acceleration"=-20.000000000000284, "jerk"=0.0, "heading"=270.0}, {"position"=399.5632346792959, "velocity"=63.65651114117066, "acceleration"=-19.999999999999574, "jerk"=7.105427357601002e-11, "heading"=270.0}, {"position"=400.1987997907076, "velocity"=63.456511141170665, "acceleration"=-19.999999999999574, "jerk"=0.0, "heading"=270.0}, {"position"=400.8323649021193, "velocity"=63.25651114117067, "acceleration"=-19.999999999999574, "jerk"=0.0, "heading"=270.0}, {"position"=401.463930013531, "velocity"=63.05651114117066, "acceleration"=-20.000000000000995, "jerk"=-1.4210854715202004e-10, "heading"=270.0}, {"position"=402.0934951249427, "velocity"=62.856511141170664, "acceleration"=-19.999999999999574, "jerk"=1.4210854715202004e-10, "heading"=270.0}, {"position"=402.7210602363544, "velocity"=62.65651114117066, "acceleration"=-20.000000000000284, "jerk"=-7.105427357601002e-11, "heading"=270.0}, {"position"=403.3466253477661, "velocity"=62.456511141170665, "acceleration"=-19.999999999999574, "jerk"=7.105427357601002e-11, "heading"=270.0}, {"position"=403.97019045917784, "velocity"=62.25651114117066, "acceleration"=-20.000000000000284, "jerk"=-7.105427357601002e-11, "heading"=270.0}, {"position"=404.59175557058956, "velocity"=62.05651114117067, "acceleration"=-19.999999999999574, "jerk"=7.105427357601002e-11, "heading"=270.0}, {"position"=405.21132068200126, "velocity"=61.856511141170664, "acceleration"=-20.000000000000284, "jerk"=-7.105427357601002e-11, "heading"=270.0}, {"position"=405.82888579341295, "velocity"=61.65651114117067, "acceleration"=-19.999999999999574, "jerk"=7.105427357601002e-11, "heading"=270.0}, {"position"=406.44445090482463, "velocity"=61.45651114117066, "acceleration"=-20.000000000000995, "jerk"=-1.4210854715202004e-10, "heading"=270.0}, {"position"=407.05801601623637, "velocity"=61.25651114117066, "acceleration"=-19.999999999999574, "jerk"=1.4210854715202004e-10, "heading"=270.0}, {"position"=407.6695811276481, "velocity"=61.05651114117066, "acceleration"=-20.000000000000284, "jerk"=-7.105427357601002e-11, "heading"=270.104960553458}, {"position"=408.2791462390598, "velocity"=60.85651114117067, "acceleration"=-19.999999999998863, "jerk"=1.4210854715202004e-10, "heading"=270.3639634543046}, {"position"=408.8867113504715, "velocity"=60.65651114117066, "acceleration"=-20.000000000000995, "jerk"=-2.1316282072803006e-10, "heading"=270.62634380295367}, {"position"=409.4922764618832, "velocity"=60.45651114117067, "acceleration"=-19.999999999998863, "jerk"=2.1316282072803006e-10, "heading"=270.89214621907075}, {"position"=410.0958415732949, "velocity"=60.25651114117068, "acceleration"=-19.999999999999574, "jerk"=-7.105427357601002e-11, "heading"=271.16143071066085}, {"position"=410.6974066847066, "velocity"=60.05651114117068, "acceleration"=-19.999999999999574, "jerk"=0.0, "heading"=271.4342360437348}, {"position"=411.2969717961183, "velocity"=59.85651114117067, "acceleration"=-20.000000000000995, "jerk"=-1.4210854715202004e-10, "heading"=271.710629680645}, {"position"=411.89453690753004, "velocity"=59.656511141170675, "acceleration"=-19.999999999999574, "jerk"=1.4210854715202004e-10, "heading"=271.99064900431364}, {"position"=412.49010201894174, "velocity"=59.45651114117067, "acceleration"=-20.000000000000284, "jerk"=-7.105427357601002e-11, "heading"=272.2743566376003}, {"position"=413.08366713035343, "velocity"=59.25651114117068, "acceleration"=-19.999999999999574, "jerk"=7.105427357601002e-11, "heading"=272.56180099422636}, {"position"=413.6752322417651, "velocity"=59.05651114117067, "acceleration"=-20.000000000000995, "jerk"=-1.4210854715202004e-10, "heading"=272.85303417502627}, {"position"=414.26479735317685, "velocity"=58.85651114117068, "acceleration"=-19.999999999998863, "jerk"=2.1316282072803006e-10, "heading"=273.14811760487174}, {"position"=414.85236246458857, "velocity"=58.656511141170675, "acceleration"=-20.000000000000284, "jerk"=-1.4210854715202004e-10, "heading"=273.44709334318907}, {"position"=415.4379275760003, "velocity"=58.45651114117068, "acceleration"=-19.999999999999574, "jerk"=7.105427357601002e-11, "heading"=273.7500294868194}, {"position"=416.021492687412, "velocity"=58.25651114117067, "acceleration"=-20.000000000000995, "jerk"=-1.4210854715202004e-10, "heading"=274.05696969875254}, {"position"=416.60305779882367, "velocity"=58.056511141170674, "acceleration"=-19.999999999999574, "jerk"=1.4210854715202004e-10, "heading"=274.36797102673825}, {"position"=417.18262291023535, "velocity"=57.85651114117067, "acceleration"=-20.000000000000284, "jerk"=-7.105427357601002e-11, "heading"=274.6830944709973}, {"position"=417.7601880216471, "velocity"=57.65651114117068, "acceleration"=-19.999999999998863, "jerk"=1.4210854715202004e-10, "heading"=275.00238342213856}, {"position"=418.3357531330588, "velocity"=57.45651114117067, "acceleration"=-20.000000000000995, "jerk"=-2.1316282072803006e-10, "heading"=275.32590470093845}, {"position"=418.9093182444705, "velocity"=57.25651114117068, "acceleration"=-19.999999999999574, "jerk"=1.4210854715202004e-10, "heading"=275.6537056516807}, {"position"=419.4808833558822, "velocity"=57.056511141170674, "acceleration"=-20.000000000000284, "jerk"=-7.105427357601002e-11, "heading"=275.98583681875607}, {"position"=420.0504484672939, "velocity"=56.85651114117067, "acceleration"=-20.000000000000284, "jerk"=0.0, "heading"=276.3223677823672}, {"position"=420.6180135787056, "velocity"=56.656511141170675, "acceleration"=-19.999999999999574, "jerk"=7.105427357601002e-11, "heading"=276.66333654242675}, {"position"=421.1835786901173, "velocity"=56.456511141170665, "acceleration"=-20.000000000000995, "jerk"=-1.4210854715202004e-10, "heading"=277.0088011027038}, {"position"=421.74714380152903, "velocity"=56.25651114117068, "acceleration"=-19.999999999998863, "jerk"=2.1316282072803006e-10, "heading"=277.3588222144209}, {"position"=422.30870891294074, "velocity"=56.056511141170674, "acceleration"=-20.000000000000284, "jerk"=-1.4210854715202004e-10, "heading"=277.7134401407597}, {"position"=422.86827402435244, "velocity"=55.85651114117068, "acceleration"=-19.999999999999574, "jerk"=7.105427357601002e-11, "heading"=278.07271319948495}, {"position"=423.42583913576414, "velocity"=55.65651114117067, "acceleration"=-20.000000000000995, "jerk"=-1.4210854715202004e-10, "heading"=278.43669574951446}, {"position"=423.9814042471758, "velocity"=55.45651114117067, "acceleration"=-19.999999999999574, "jerk"=1.4210854715202004e-10, "heading"=278.80542775074684}, {"position"=424.53496935858755, "velocity"=55.25651114117067, "acceleration"=-20.000000000000284, "jerk"=-7.105427357601002e-11, "heading"=279.17896504913665}, {"position"=425.08653446999926, "velocity"=55.05651114117068, "acceleration"=-19.999999999998863, "jerk"=1.4210854715202004e-10, "heading"=279.557358111336}, {"position"=425.636099581411, "velocity"=54.85651114117067, "acceleration"=-20.000000000000995, "jerk"=-2.1316282072803006e-10, "heading"=279.9406437476047}, {"position"=426.1836646928227, "velocity"=54.656511141170675, "acceleration"=-19.999999999999574, "jerk"=1.4210854715202004e-10, "heading"=280.3288723274611}, {"position"=426.72922980423436, "velocity"=54.45651114117067, "acceleration"=-20.000000000000284, "jerk"=-7.105427357601002e-11, "heading"=280.72209286960975}, {"position"=427.27279491564605, "velocity"=54.25651114117068, "acceleration"=-19.999999999999574, "jerk"=7.105427357601002e-11, "heading"=281.120335951735}, {"position"=427.8143600270578, "velocity"=54.05651114117067, "acceleration"=-20.000000000000995, "jerk"=-1.4210854715202004e-10, "heading"=281.5236433084465}, {"position"=428.3539251384695, "velocity"=53.85651114117068, "acceleration"=-19.999999999998863, "jerk"=2.1316282072803006e-10, "heading"=281.9320647527151}, {"position"=428.8914902498812, "velocity"=53.656511141170675, "acceleration"=-20.000000000000284, "jerk"=-1.4210854715202004e-10, "heading"=282.345621374788}, {"position"=429.4270553612929, "velocity"=53.45651114117068, "acceleration"=-19.999999999999574, "jerk"=7.105427357601002e-11, "heading"=282.7643460476821}, {"position"=429.9606204727046, "velocity"=53.25651114117067, "acceleration"=-20.000000000000995, "jerk"=-1.4210854715202004e-10, "heading"=283.18828225239554}, {"position"=430.49218558411627, "velocity"=53.056511141170674, "acceleration"=-19.999999999999574, "jerk"=1.4210854715202004e-10, "heading"=283.6174472480843}, {"position"=431.021750695528, "velocity"=52.85651114117067, "acceleration"=-20.000000000000284, "jerk"=-7.105427357601002e-11, "heading"=284.05186244447606}, {"position"=431.5493158069397, "velocity"=52.656511141170675, "acceleration"=-19.999999999999574, "jerk"=7.105427357601002e-11, "heading"=284.4915555633204}, {"position"=432.0748809183514, "velocity"=52.45651114117067, "acceleration"=-20.000000000000284, "jerk"=-7.105427357601002e-11, "heading"=284.93654745454484}, {"position"=432.5984460297631, "velocity"=52.25651114117068, "acceleration"=-19.999999999999574, "jerk"=7.105427357601002e-11, "heading"=285.3868426615331}, {"position"=433.1200111411748, "velocity"=52.056511141170674, "acceleration"=-20.000000000000284, "jerk"=-7.105427357601002e-11, "heading"=285.84245144653823}, {"position"=433.6395762525865, "velocity"=51.85651114117068, "acceleration"=-19.999999999999574, "jerk"=7.105427357601002e-11, "heading"=286.3033947679342}, {"position"=434.1571413639982, "velocity"=51.65651114117067, "acceleration"=-20.000000000000995, "jerk"=-1.4210854715202004e-10, "heading"=286.76966105386055}, {"position"=434.67270647540994, "velocity"=51.45651114117067, "acceleration"=-19.999999999999574, "jerk"=1.4210854715202004e-10, "heading"=287.24124637717824}, {"position"=435.18627158682165, "velocity"=51.25651114117068, "acceleration"=-19.999999999999574, "jerk"=0.0, "heading"=287.7181496624582}, {"position"=435.69783669823335, "velocity"=51.05651114117068, "acceleration"=-19.999999999999574, "jerk"=0.0, "heading"=288.20036200422766}, {"position"=436.20740180964503, "velocity"=50.85651114117067, "acceleration"=-20.000000000000995, "jerk"=-1.4210854715202004e-10, "heading"=288.6878561017957}, {"position"=436.7149669210567, "velocity"=50.656511141170675, "acceleration"=-19.999999999999574, "jerk"=1.4210854715202004e-10, "heading"=289.18060899151055}, {"position"=437.22053203246844, "velocity"=50.45651114117067, "acceleration"=-20.000000000000284, "jerk"=-7.105427357601002e-11, "heading"=289.6786061101804}, {"position"=437.72409714388016, "velocity"=50.25651114117068, "acceleration"=-19.999999999999574, "jerk"=7.105427357601002e-11, "heading"=290.1818010661012}, {"position"=438.22566225529187, "velocity"=50.05651114117067, "acceleration"=-20.000000000000995, "jerk"=-1.4210854715202004e-10, "heading"=290.6901512611895}, {"position"=438.72522736670356, "velocity"=49.85651114117068, "acceleration"=-19.999999999998863, "jerk"=2.1316282072803006e-10, "heading"=291.2036165173339}, {"position"=439.22279247811525, "velocity"=49.656511141170675, "acceleration"=-20.000000000000284, "jerk"=-1.4210854715202004e-10, "heading"=291.72214678621594}, {"position"=439.71835758952693, "velocity"=49.45651114117068, "acceleration"=-19.999999999999574, "jerk"=7.105427357601002e-11, "heading"=292.24567251132873}, {"position"=440.21192270093866, "velocity"=49.25651114117067, "acceleration"=-20.000000000000995, "jerk"=-1.4210854715202004e-10, "heading"=292.77412780292946}, {"position"=440.7034878123504, "velocity"=49.056511141170674, "acceleration"=-19.999999999999574, "jerk"=1.4210854715202004e-10, "heading"=293.30745422462536}, {"position"=441.1930529237621, "velocity"=48.85651114117067, "acceleration"=-20.000000000000284, "jerk"=-7.105427357601002e-11, "heading"=293.84555528585486}, {"position"=441.6806180351738, "velocity"=48.65651114117068, "acceleration"=-19.999999999998863, "jerk"=1.4210854715202004e-10, "heading"=294.38834319470476}, {"position"=442.16618314658547, "velocity"=48.45651114117067, "acceleration"=-20.000000000000995, "jerk"=-2.1316282072803006e-10, "heading"=294.93573671059465}, {"position"=442.64974825799715, "velocity"=48.25651114117068, "acceleration"=-19.999999999999574, "jerk"=1.4210854715202004e-10, "heading"=295.48762220917814}, {"position"=443.1313133694089, "velocity"=48.056511141170674, "acceleration"=-20.000000000000284, "jerk"=-7.105427357601002e-11, "heading"=296.0438869267255}, {"position"=443.6108784808206, "velocity"=47.85651114117067, "acceleration"=-20.000000000000284, "jerk"=0.0, "heading"=296.6044268491836}, {"position"=444.0884435922323, "velocity"=47.656511141170675, "acceleration"=-19.999999999999574, "jerk"=7.105427357601002e-11, "heading"=297.1691070628833}, {"position"=444.564008703644, "velocity"=47.456511141170665, "acceleration"=-20.000000000000995, "jerk"=-1.4210854715202004e-10, "heading"=297.73779173050497}, {"position"=445.0375738150557, "velocity"=47.25651114117068, "acceleration"=-19.999999999998863, "jerk"=2.1316282072803006e-10, "heading"=298.310357040823}, {"position"=445.5091389264674, "velocity"=47.05651114117069, "acceleration"=-19.999999999998863, "jerk"=0.0, "heading"=298.88664067992033}, {"position"=445.97870403787914, "velocity"=46.85651114117068, "acceleration"=-20.000000000000995, "jerk"=-2.1316282072803006e-10, "heading"=299.46649208985616}, {"position"=446.44626914929086, "velocity"=46.65651114117068, "acceleration"=-19.999999999999574, "jerk"=1.4210854715202004e-10, "heading"=300.04975713086316}, {"position"=446.91183426070256, "velocity"=46.45651114117068, "acceleration"=-20.000000000000284, "jerk"=-7.105427357601002e-11, "heading"=300.6362550639972}, {"position"=447.37539937211426, "velocity"=46.25651114117068, "acceleration"=-20.000000000000284, "jerk"=0.0, "heading"=301.22582405583637}, {"position"=447.83696448352595, "velocity"=46.05651114117068, "acceleration"=-19.999999999999574, "jerk"=7.105427357601002e-11, "heading"=301.8182722536213}, {"position"=448.2965295949377, "velocity"=45.85651114117067, "acceleration"=-20.000000000000995, "jerk"=-1.4210854715202004e-10, "heading"=302.4134162440037}, {"position"=448.7540947063494, "velocity"=45.65651114117068, "acceleration"=-19.999999999998863, "jerk"=2.1316282072803006e-10, "heading"=303.01106246573283}, {"position"=449.2096598177611, "velocity"=45.45651114117068, "acceleration"=-20.000000000000284, "jerk"=-1.4210854715202004e-10, "heading"=303.6110079347656}, {"position"=449.6632249291728, "velocity"=45.256511141170684, "acceleration"=-19.999999999999574, "jerk"=7.105427357601002e-11, "heading"=304.2130533081122}, {"position"=450.1147900405845, "velocity"=45.056511141170674, "acceleration"=-20.000000000000995, "jerk"=-1.4210854715202004e-10, "heading"=304.8169824752847}, {"position"=450.5643551519962, "velocity"=44.85651114117068, "acceleration"=-19.999999999999574, "jerk"=1.4210854715202004e-10, "heading"=305.42258714898213}, {"position"=451.01192026340794, "velocity"=44.656511141170675, "acceleration"=-20.000000000000284, "jerk"=-7.105427357601002e-11, "heading"=306.0296439255259}, {"position"=451.45748537481967, "velocity"=44.45651114117069, "acceleration"=-19.999999999998863, "jerk"=1.4210854715202004e-10, "heading"=306.6379336520938}, {"position"=451.9010504862314, "velocity"=44.25651114117068, "acceleration"=-20.000000000000995, "jerk"=-2.1316282072803006e-10, "heading"=307.24723046603344}, {"position"=452.3426155976431, "velocity"=44.05651114117068, "acceleration"=-19.999999999999574, "jerk"=1.4210854715202004e-10, "heading"=307.85730401414054}, {"position"=452.7821807090548, "velocity"=43.85651114117068, "acceleration"=-20.000000000000284, "jerk"=-7.105427357601002e-11, "heading"=308.467929395661}, {"position"=453.21974582046647, "velocity"=43.65651114117068, "acceleration"=-19.999999999999574, "jerk"=7.105427357601002e-11, "heading"=309.0788692086994}, {"position"=453.6553109318782, "velocity"=43.45651114117067, "acceleration"=-20.000000000000995, "jerk"=-1.4210854715202004e-10, "heading"=309.68989344251787}, {"position"=454.08887604328993, "velocity"=43.25651114117068, "acceleration"=-19.999999999999574, "jerk"=1.4210854715202004e-10, "heading"=310.30076861512566}, {"position"=454.52044115470164, "velocity"=43.05651114117068, "acceleration"=-19.999999999999574, "jerk"=0.0, "heading"=310.91125948633163}, {"position"=454.95000626611335, "velocity"=42.856511141170685, "acceleration"=-19.999999999999574, "jerk"=0.0, "heading"=311.5211338842268}, {"position"=455.37757137752504, "velocity"=42.656511141170675, "acceleration"=-20.000000000000995, "jerk"=-1.4210854715202004e-10, "heading"=312.13016015290594}, {"position"=455.80313648893673, "velocity"=42.45651114117068, "acceleration"=-19.999999999999574, "jerk"=1.4210854715202004e-10, "heading"=312.73810683888007}, {"position"=456.22670160034846, "velocity"=42.25651114117068, "acceleration"=-20.000000000000284, "jerk"=-7.105427357601002e-11, "heading"=313.34474583965715}, {"position"=456.6482667117602, "velocity"=42.05651114117068, "acceleration"=-19.999999999999574, "jerk"=7.105427357601002e-11, "heading"=313.9498514938354}, {"position"=457.0678318231719, "velocity"=41.85651114117068, "acceleration"=-20.000000000000284, "jerk"=-7.105427357601002e-11, "heading"=314.5532005175991}, {"position"=457.4853969345836, "velocity"=41.65651114117068, "acceleration"=-19.999999999999574, "jerk"=7.105427357601002e-11, "heading"=315.15457324245574}, {"position"=457.9009620459953, "velocity"=41.45651114117068, "acceleration"=-20.000000000000284, "jerk"=-7.105427357601002e-11, "heading"=315.7537550482761}, {"position"=458.314527157407, "velocity"=41.256511141170684, "acceleration"=-19.999999999999574, "jerk"=7.105427357601002e-11, "heading"=316.3505352020104}, {"position"=458.7260922688187, "velocity"=41.056511141170674, "acceleration"=-20.000000000000995, "jerk"=-1.4210854715202004e-10, "heading"=316.9447078113313}, {"position"=459.13565738023044, "velocity"=40.85651114117068, "acceleration"=-19.999999999999574, "jerk"=1.4210854715202004e-10, "heading"=317.53607224157287}, {"position"=459.54322249164215, "velocity"=40.656511141170675, "acceleration"=-20.000000000000284, "jerk"=-7.105427357601002e-11, "heading"=318.12443350757627}, {"position"=459.94878760305386, "velocity"=40.45651114117069, "acceleration"=-19.999999999998863, "jerk"=1.4210854715202004e-10, "heading"=318.70960263874395}, {"position"=460.35235271446555, "velocity"=40.256511141170684, "acceleration"=-20.000000000000284, "jerk"=-1.4210854715202004e-10, "heading"=319.2913970158396}, {"position"=460.75391782587724, "velocity"=40.05651114117069, "acceleration"=-19.999999999999574, "jerk"=7.105427357601002e-11, "heading"=319.8696406783121}, {"position"=461.15348293728897, "velocity"=39.856511141170685, "acceleration"=-20.000000000000284, "jerk"=-7.105427357601002e-11, "heading"=320.4441646011697}, {"position"=461.5510480487007, "velocity"=39.65651114117069, "acceleration"=-19.999999999999574, "jerk"=7.105427357601002e-11, "heading"=321.0148027645164}, {"position"=461.9466131601124, "velocity"=39.45651114117068, "acceleration"=-20.000000000000995, "jerk"=-1.4210854715202004e-10, "heading"=321.5814011117995}, {"position"=462.3401782715241, "velocity"=39.256511141170684, "acceleration"=-19.999999999999574, "jerk"=1.4210854715202004e-10, "heading"=322.14381426090955}, {"position"=462.7317433829358, "velocity"=39.05651114117068, "acceleration"=-20.000000000000284, "jerk"=-7.105427357601002e-11, "heading"=322.70190283232773}, {"position"=463.1213084943475, "velocity"=38.85651114117069, "acceleration"=-19.999999999998863, "jerk"=1.4210854715202004e-10, "heading"=323.25553092029844}, {"position"=463.5088736057592, "velocity"=38.65651114117068, "acceleration"=-20.000000000000995, "jerk"=-2.1316282072803006e-10, "heading"=323.8045677236461}, {"position"=463.89443871717094, "velocity"=38.45651114117069, "acceleration"=-19.999999999999574, "jerk"=1.4210854715202004e-10, "heading"=324.3489060158224}, {"position"=464.27800382858265, "velocity"=38.256511141170684, "acceleration"=-20.000000000000284, "jerk"=-7.105427357601002e-11, "heading"=324.88842891365164}, {"position"=464.65956893999436, "velocity"=38.05651114117069, "acceleration"=-19.999999999999574, "jerk"=7.105427357601002e-11, "heading"=325.42303112422775}, {"position"=465.03913405140605, "velocity"=37.85651114117068, "acceleration"=-20.000000000000995, "jerk"=-1.4210854715202004e-10, "heading"=325.9526283642025}, {"position"=465.41669916281774, "velocity"=37.65651114117069, "acceleration"=-19.999999999998863, "jerk"=2.1316282072803006e-10, "heading"=326.4771141191666}, {"position"=465.79226427422947, "velocity"=37.45651114117069, "acceleration"=-20.000000000000284, "jerk"=-1.4210854715202004e-10, "heading"=326.9964290842288}, {"position"=466.1658293856412, "velocity"=37.25651114117069, "acceleration"=-19.999999999999574, "jerk"=7.105427357601002e-11, "heading"=327.51047896304135}, {"position"=466.5373944970529, "velocity"=37.05651114117068, "acceleration"=-20.000000000000995, "jerk"=-1.4210854715202004e-10, "heading"=328.01921369068384}, {"position"=466.9069596084646, "velocity"=36.856511141170685, "acceleration"=-19.999999999999574, "jerk"=1.4210854715202004e-10, "heading"=328.5225679310066}, {"position"=467.2745247198763, "velocity"=36.65651114117069, "acceleration"=-19.999999999999574, "jerk"=0.0, "heading"=329.02048160809994}, {"position"=467.640089831288, "velocity"=36.456511141170694, "acceleration"=-19.999999999999574, "jerk"=0.0, "heading"=329.51292202077053}, {"position"=468.0036549426997, "velocity"=36.256511141170684, "acceleration"=-20.000000000000995, "jerk"=-1.4210854715202004e-10, "heading"=329.99984507844323}, {"position"=468.36522005411143, "velocity"=36.05651114117069, "acceleration"=-19.999999999999574, "jerk"=1.4210854715202004e-10, "heading"=330.4812033882082}, {"position"=468.72478516552314, "velocity"=35.85651114117069, "acceleration"=-19.999999999999574, "jerk"=0.0, "heading"=330.9569839244473}, {"position"=469.08235027693485, "velocity"=35.65651114117069, "acceleration"=-20.000000000000284, "jerk"=-7.105427357601002e-11, "heading"=331.4271633604797}, {"position"=469.43791538834654, "velocity"=35.456511141170694, "acceleration"=-19.999999999999574, "jerk"=7.105427357601002e-11, "heading"=331.89172404718244}, {"position"=469.7914804997582, "velocity"=35.25651114117069, "acceleration"=-20.000000000000284, "jerk"=-7.105427357601002e-11, "heading"=332.35065382354867}, {"position"=470.14304561116995, "velocity"=35.05651114117069, "acceleration"=-20.000000000000284, "jerk"=0.0, "heading"=332.8039458217977}, {"position"=470.4926107225817, "velocity"=34.856511141170685, "acceleration"=-20.000000000000284, "jerk"=0.0, "heading"=333.2515982681019}, {"position"=470.8401758339934, "velocity"=34.6565111411707, "acceleration"=-19.999999999998863, "jerk"=1.4210854715202004e-10, "heading"=333.6936142799466}, {"position"=471.1857409454051, "velocity"=34.456511141170694, "acceleration"=-20.000000000000284, "jerk"=-1.4210854715202004e-10, "heading"=334.1300016610876}, {"position"=471.5293060568168, "velocity"=34.25651114117069, "acceleration"=-20.000000000000284, "jerk"=0.0, "heading"=334.5607726950145}, {"position"=471.87087116822846, "velocity"=34.05651114117069, "acceleration"=-20.000000000000284, "jerk"=0.0, "heading"=334.98594393777324}, {"position"=472.2104362796402, "velocity"=33.856511141170685, "acceleration"=-20.000000000000284, "jerk"=0.0, "heading"=335.4055360109425}, {"position"=472.5480013910519, "velocity"=33.6565111411707, "acceleration"=-19.999999999998863, "jerk"=1.4210854715202004e-10, "heading"=335.8195733955005}, {"position"=472.8835665024636, "velocity"=33.456511141170694, "acceleration"=-20.000000000000284, "jerk"=-1.4210854715202004e-10, "heading"=336.228084227262}, {"position"=473.2171316138753, "velocity"=33.25651114117069, "acceleration"=-20.000000000000284, "jerk"=0.0, "heading"=336.6310869364625}, {"position"=473.548696725287, "velocity"=33.056511141170695, "acceleration"=-19.999999999999574, "jerk"=7.105427357601002e-11, "heading"=337.02861634053585}, {"position"=473.8782618366987, "velocity"=32.8565111411707, "acceleration"=-19.999999999999574, "jerk"=0.0, "heading"=337.4207198864475}, {"position"=474.2058269481104, "velocity"=32.6565111411707, "acceleration"=-20.000000000000284, "jerk"=-7.105427357601002e-11, "heading"=337.80742797223434}, {"position"=474.53139205952215, "velocity"=32.456511141170694, "acceleration"=-20.000000000000284, "jerk"=0.0, "heading"=338.1887682106313}, {"position"=474.85495717093386, "velocity"=32.25651114117069, "acceleration"=-20.000000000000284, "jerk"=0.0, "heading"=338.5648088427341}, {"position"=475.17652228234556, "velocity"=32.0565111411707, "acceleration"=-19.999999999998863, "jerk"=1.4210854715202004e-10, "heading"=338.93556208342335}, {"position"=475.49608739375725, "velocity"=31.856511141170696, "acceleration"=-20.00000000000064, "jerk"=-1.7763568394002505e-10, "heading"=339.30110330917256}, {"position"=475.81365250516893, "velocity"=31.656511141170697, "acceleration"=-19.99999999999993, "jerk"=7.105427357601002e-11, "heading"=339.6614543581399}, {"position"=476.12921761658066, "velocity"=31.456511141170697, "acceleration"=-19.99999999999993, "jerk"=0.0, "heading"=340.0166907937528}, {"position"=476.4427827279924, "velocity"=31.256511141170698, "acceleration"=-19.99999999999993, "jerk"=0.0, "heading"=340.36682879453014}, {"position"=476.7543478394041, "velocity"=31.056511141170695, "acceleration"=-20.000000000000284, "jerk"=-3.552713678800501e-11, "heading"=340.71195351640966}, {"position"=477.0639129508158, "velocity"=30.856511141170703, "acceleration"=-19.99999999999922, "jerk"=1.0658141036401503e-10, "heading"=341.05209542811076}, {"position"=477.3714780622275, "velocity"=30.6565111411707, "acceleration"=-20.000000000000284, "jerk"=-1.0658141036401503e-10, "heading"=341.38731043714233}, {"position"=477.67704317363916, "velocity"=30.456511141170704, "acceleration"=-19.999999999999574, "jerk"=7.105427357601002e-11, "heading"=341.71766504134985}, {"position"=477.9806082850509, "velocity"=30.2565111411707, "acceleration"=-20.000000000000284, "jerk"=-7.105427357601002e-11, "heading"=342.0432078988646}, {"position"=478.2821733964626, "velocity"=30.056511141170702, "acceleration"=-19.99999999999993, "jerk"=3.552713678800501e-11, "heading"=342.36397716071747}, {"position"=478.5817385078743, "velocity"=29.8565111411707, "acceleration"=-20.000000000000284, "jerk"=-3.552713678800501e-11, "heading"=342.68004776625935}, {"position"=478.879303619286, "velocity"=29.656511141170704, "acceleration"=-19.999999999999574, "jerk"=7.105427357601002e-11, "heading"=342.99147411473564}, {"position"=479.1748687306977, "velocity"=29.4565111411707, "acceleration"=-20.000000000000284, "jerk"=-7.105427357601002e-11, "heading"=343.29831118899693}, {"position"=479.4684338421094, "velocity"=29.2565111411707, "acceleration"=-19.99999999999993, "jerk"=3.552713678800501e-11, "heading"=343.6006144722321}, {"position"=479.7599989535211, "velocity"=29.056511141170702, "acceleration"=-19.99999999999993, "jerk"=0.0, "heading"=343.89843986875087}, {"position"=480.04956406493284, "velocity"=28.856511141170703, "acceleration"=-19.99999999999993, "jerk"=0.0, "heading"=344.19184362872375}, {"position"=480.33712917634455, "velocity"=28.656511141170707, "acceleration"=-19.999999999999574, "jerk"=3.552713678800501e-11, "heading"=344.4808822767833}, {"position"=480.62269428775625, "velocity"=28.456511141170708, "acceleration"=-19.99999999999993, "jerk"=-3.552713678800501e-11, "heading"=344.76561254438343}, {"position"=480.90625939916794, "velocity"=28.256511141170705, "acceleration"=-20.000000000000284, "jerk"=-3.552713678800501e-11, "heading"=345.0460913058119}, {"position"=481.1878245105796, "velocity"=28.05651114117071, "acceleration"=-19.999999999999574, "jerk"=7.105427357601002e-11, "heading"=345.3223755177454}, {"position"=481.46738962199134, "velocity"=27.856511141170706, "acceleration"=-20.000000000000284, "jerk"=-7.105427357601002e-11, "heading"=345.5945221622374}, {"position"=481.74495473340306, "velocity"=27.656511141170707, "acceleration"=-19.99999999999993, "jerk"=3.552713678800501e-11, "heading"=345.8625881930236}, {"position"=482.02051984481477, "velocity"=27.456511141170708, "acceleration"=-19.99999999999993, "jerk"=0.0, "heading"=346.126630485032}, {"position"=482.29408495622647, "velocity"=27.25651114117071, "acceleration"=-19.99999999999993, "jerk"=0.0, "heading"=346.38670578698253}, {"position"=482.56565006763816, "velocity"=27.056511141170706, "acceleration"=-20.000000000000284, "jerk"=-3.552713678800501e-11, "heading"=346.64285603453857}, {"position"=482.83521517904984, "velocity"=26.85651114117071, "acceleration"=-19.999999999999574, "jerk"=7.105427357601002e-11, "heading"=346.895140331819}, {"position"=483.10278029046157, "velocity"=26.65651114117071, "acceleration"=-19.99999999999993, "jerk"=-3.552713678800501e-11, "heading"=347.14362382471234}, {"position"=483.3683454018733, "velocity"=26.456511141170715, "acceleration"=-19.999999999999574, "jerk"=3.552713678800501e-11, "heading"=347.3883605263655}, {"position"=483.631910513285, "velocity"=26.256511141170712, "acceleration"=-20.000000000000284, "jerk"=-7.105427357601002e-11, "heading"=347.62937460464383}, {"position"=483.8934756246967, "velocity"=26.056511141170713, "acceleration"=-19.99999999999993, "jerk"=3.552713678800501e-11, "heading"=347.8667516688963}, {"position"=484.1530407361084, "velocity"=25.856511141170714, "acceleration"=-19.99999999999993, "jerk"=0.0, "heading"=348.100532060787}, {"position"=484.41060584752006, "velocity"=25.656511141170714, "acceleration"=-19.99999999999993, "jerk"=0.0, "heading"=348.33075587646044}, {"position"=484.6661709589318, "velocity"=25.45651114117071, "acceleration"=-20.000000000000284, "jerk"=-3.552713678800501e-11, "heading"=348.5575000449887}, {"position"=484.9197360703435, "velocity"=25.256511141170712, "acceleration"=-19.99999999999993, "jerk"=3.552713678800501e-11, "heading"=348.7807758702239}, {"position"=485.1713011817552, "velocity"=25.056511141170713, "acceleration"=-19.99999999999993, "jerk"=0.0, "heading"=349.0006764829036}, {"position"=485.4208662931669, "velocity"=24.856511141170714, "acceleration"=-19.99999999999993, "jerk"=0.0, "heading"=349.217206268733}, {"position"=485.6684314045786, "velocity"=24.65651114117071, "acceleration"=-20.000000000000284, "jerk"=-3.552713678800501e-11, "heading"=349.4304527513581}, {"position"=485.9139965159903, "velocity"=24.456511141170715, "acceleration"=-19.999999999999574, "jerk"=7.105427357601002e-11, "heading"=349.6404348622633}, {"position"=486.157561627402, "velocity"=24.256511141170712, "acceleration"=-20.000000000000284, "jerk"=-7.105427357601002e-11, "heading"=349.84721315662324}, {"position"=486.3991267388137, "velocity"=24.056511141170716, "acceleration"=-19.999999999999574, "jerk"=7.105427357601002e-11, "heading"=350.0508421389383}, {"position"=486.6386918502254, "velocity"=23.856511141170714, "acceleration"=-20.000000000000284, "jerk"=-7.105427357601002e-11, "heading"=350.25133450376177}, {"position"=486.8762569616371, "velocity"=23.656511141170718, "acceleration"=-19.999999999999574, "jerk"=7.105427357601002e-11, "heading"=350.44876624738527}, {"position"=487.1118220730488, "velocity"=23.456511141170715, "acceleration"=-20.000000000000284, "jerk"=-7.105427357601002e-11, "heading"=350.6431788945923}, {"position"=487.34538718446055, "velocity"=23.256511141170712, "acceleration"=-20.000000000000284, "jerk"=0.0, "heading"=350.8345951790319}, {"position"=487.5769522958723, "velocity"=23.056511141170716, "acceleration"=-19.999999999999574, "jerk"=7.105427357601002e-11, "heading"=351.0230697679119}, {"position"=487.806517407284, "velocity"=22.856511141170714, "acceleration"=-20.000000000000284, "jerk"=-7.105427357601002e-11, "heading"=351.2086496249362}, {"position"=488.0340825186957, "velocity"=22.65651114117071, "acceleration"=-20.000000000000284, "jerk"=0.0, "heading"=351.3913743898024}, {"position"=488.2596476301074, "velocity"=22.456511141170715, "acceleration"=-19.999999999999574, "jerk"=7.105427357601002e-11, "heading"=351.57128322826753}, {"position"=488.4832127415191, "velocity"=22.256511141170712, "acceleration"=-20.000000000000284, "jerk"=-7.105427357601002e-11, "heading"=351.7484067784427}, {"position"=488.7047778529308, "velocity"=22.056511141170713, "acceleration"=-19.99999999999993, "jerk"=3.552713678800501e-11, "heading"=351.9227890122941}, {"position"=488.92434296434254, "velocity"=21.85651114117071, "acceleration"=-20.000000000000284, "jerk"=-3.552713678800501e-11, "heading"=352.0944723563072}, {"position"=489.14190807575426, "velocity"=21.656511141170714, "acceleration"=-19.999999999999574, "jerk"=7.105427357601002e-11, "heading"=352.263494031858}, {"position"=489.35747318716597, "velocity"=21.45651114117071, "acceleration"=-20.000000000000284, "jerk"=-7.105427357601002e-11, "heading"=352.42989077948556}, {"position"=489.57103829857766, "velocity"=21.256511141170712, "acceleration"=-19.99999999999993, "jerk"=3.552713678800501e-11, "heading"=352.59369885907165}, {"position"=489.78260340998935, "velocity"=21.056511141170713, "acceleration"=-19.99999999999993, "jerk"=0.0, "heading"=352.75495405046036}, {"position"=489.9921685214011, "velocity"=20.856511141170714, "acceleration"=-19.99999999999993, "jerk"=0.0, "heading"=352.91369165448964}, {"position"=490.1997336328128, "velocity"=20.65651114117071, "acceleration"=-20.000000000000284, "jerk"=-3.552713678800501e-11, "heading"=353.0699464944055}, {"position"=490.4052987442245, "velocity"=20.456511141170715, "acceleration"=-19.999999999999574, "jerk"=7.105427357601002e-11, "heading"=353.2237529176333}, {"position"=490.60886385563623, "velocity"=20.256511141170712, "acceleration"=-20.000000000000284, "jerk"=-7.105427357601002e-11, "heading"=353.37514479787956}, {"position"=490.8104289670479, "velocity"=20.056511141170713, "acceleration"=-19.99999999999993, "jerk"=3.552713678800501e-11, "heading"=353.5241497954468}, {"position"=491.0099940784596, "velocity"=19.856511141170714, "acceleration"=-19.99999999999993, "jerk"=0.0, "heading"=353.67079778546076}, {"position"=491.20755918987135, "velocity"=19.656511141170714, "acceleration"=-19.99999999999993, "jerk"=0.0, "heading"=353.81512794266933}, {"position"=491.40312430128307, "velocity"=19.45651114117071, "acceleration"=-20.000000000000284, "jerk"=-3.552713678800501e-11, "heading"=353.9571722997996}, {"position"=491.5966894126948, "velocity"=19.256511141170716, "acceleration"=-19.999999999999574, "jerk"=7.105427357601002e-11, "heading"=354.09696243027776}, {"position"=491.7882545241065, "velocity"=19.056511141170713, "acceleration"=-20.000000000000284, "jerk"=-7.105427357601002e-11, "heading"=354.23452523877233}, {"position"=491.9778196355182, "velocity"=18.856511141170714, "acceleration"=-19.99999999999993, "jerk"=3.552713678800501e-11, "heading"=354.36987486636616}, {"position"=492.1653847469299, "velocity"=18.656511141170714, "acceleration"=-19.99999999999993, "jerk"=0.0, "heading"=354.50306030641076}, {"position"=492.3509498583416, "velocity"=18.456511141170715, "acceleration"=-19.99999999999993, "jerk"=0.0, "heading"=354.6341113587482}, {"position"=492.53451496975333, "velocity"=18.256511141170716, "acceleration"=-19.99999999999993, "jerk"=0.0, "heading"=354.76303577001704}, {"position"=492.71608008116505, "velocity"=18.056511141170713, "acceleration"=-20.000000000000284, "jerk"=-3.552713678800501e-11, "heading"=354.88987283732524}, {"position"=492.89564519257675, "velocity"=17.856511141170714, "acceleration"=-19.99999999999993, "jerk"=3.552713678800501e-11, "heading"=355.01466043257705}, {"position"=493.07321030398845, "velocity"=17.65651114117071, "acceleration"=-20.000000000000284, "jerk"=-3.552713678800501e-11, "heading"=355.1373943572271}, {"position"=493.24877541540013, "velocity"=17.45651114117071, "acceleration"=-19.99999999999993, "jerk"=3.552713678800501e-11, "heading"=355.25812828571844}, {"position"=493.42234052681187, "velocity"=17.256511141170712, "acceleration"=-19.99999999999993, "jerk"=0.0, "heading"=355.37687576667037}, {"position"=493.5939056382236, "velocity"=17.05651114117071, "acceleration"=-20.000000000000284, "jerk"=-3.552713678800501e-11, "heading"=355.49365771868537}, {"position"=493.7634707496353, "velocity"=16.85651114117071, "acceleration"=-19.99999999999993, "jerk"=3.552713678800501e-11, "heading"=355.60851099417795}, {"position"=493.931035861047, "velocity"=16.65651114117071, "acceleration"=-19.99999999999993, "jerk"=0.0, "heading"=355.7214396542129}, {"position"=494.0966009724587, "velocity"=16.45651114117071, "acceleration"=-19.99999999999993, "jerk"=0.0, "heading"=355.83248817618045}, {"position"=494.2601660838704, "velocity"=16.256511141170712, "acceleration"=-19.99999999999993, "jerk"=0.0, "heading"=355.94165929129997}, {"position"=494.4217311952821, "velocity"=16.056511141170713, "acceleration"=-19.99999999999993, "jerk"=0.0, "heading"=356.04898978795626}, {"position"=494.58129630669384, "velocity"=15.85651114117071, "acceleration"=-20.000000000000284, "jerk"=-3.552713678800501e-11, "heading"=356.1544962374381}, {"position"=494.73886141810556, "velocity"=15.65651114117071, "acceleration"=-19.99999999999993, "jerk"=3.552713678800501e-11, "heading"=356.25819277699907}, {"position"=494.89442652951726, "velocity"=15.45651114117071, "acceleration"=-20.000000000000107, "jerk"=-1.7763568394002505e-11, "heading"=356.3601203828808}, {"position"=495.04799164092896, "velocity"=15.25651114117071, "acceleration"=-19.99999999999993, "jerk"=1.7763568394002505e-11, "heading"=356.4602686980067}, {"position"=495.19955675234064, "velocity"=15.056511141170711, "acceleration"=-19.99999999999993, "jerk"=0.0, "heading"=356.55868173750946}, {"position"=495.3491218637524, "velocity"=14.856511141170712, "acceleration"=-19.99999999999993, "jerk"=0.0, "heading"=356.6553813051004}, {"position"=495.4966869751641, "velocity"=14.656511141170713, "acceleration"=-19.99999999999993, "jerk"=0.0, "heading"=356.75036006233665}, {"position"=495.6422520865758, "velocity"=14.456511141170713, "acceleration"=-19.99999999999993, "jerk"=0.0, "heading"=356.8436589510187}, {"position"=495.7858171979875, "velocity"=14.256511141170712, "acceleration"=-20.000000000000107, "jerk"=-1.7763568394002505e-11, "heading"=356.93529722024044}, {"position"=495.9273823093992, "velocity"=14.056511141170713, "acceleration"=-19.99999999999993, "jerk"=1.7763568394002505e-11, "heading"=357.0252864590709}, {"position"=496.0669474208109, "velocity"=13.856511141170712, "acceleration"=-20.000000000000107, "jerk"=-1.7763568394002505e-11, "heading"=357.1136326418222}, {"position"=496.2045125322226, "velocity"=13.65651114117071, "acceleration"=-20.000000000000107, "jerk"=0.0, "heading"=357.2003685464869}, {"position"=496.34007764363434, "velocity"=13.456511141170708, "acceleration"=-20.000000000000284, "jerk"=-1.7763568394002505e-11, "heading"=357.2855098156728}, {"position"=496.47364275504606, "velocity"=13.256511141170709, "acceleration"=-19.99999999999993, "jerk"=3.552713678800501e-11, "heading"=357.3690718392881}, {"position"=496.60520786645776, "velocity"=13.056511141170708, "acceleration"=-20.000000000000107, "jerk"=-1.7763568394002505e-11, "heading"=357.4510697576821}, {"position"=496.73477297786945, "velocity"=12.856511141170708, "acceleration"=-19.99999999999993, "jerk"=1.7763568394002505e-11, "heading"=357.53150990122293}, {"position"=496.86233808928114, "velocity"=12.656511141170709, "acceleration"=-19.99999999999993, "jerk"=0.0, "heading"=357.61041455959884}, {"position"=496.98790320069287, "velocity"=12.456511141170708, "acceleration"=-20.000000000000107, "jerk"=-1.7763568394002505e-11, "heading"=357.6878007717818}, {"position"=497.1114683121046, "velocity"=12.256511141170709, "acceleration"=-19.99999999999993, "jerk"=1.7763568394002505e-11, "heading"=357.76368269489234}, {"position"=497.2330334235163, "velocity"=12.05651114117071, "acceleration"=-19.99999999999993, "jerk"=0.0, "heading"=357.8380742523415}, {"position"=497.352598534928, "velocity"=11.856511141170708, "acceleration"=-20.000000000000107, "jerk"=-1.7763568394002505e-11, "heading"=357.9109891368511}, {"position"=497.4701636463397, "velocity"=11.656511141170709, "acceleration"=-19.99999999999993, "jerk"=1.7763568394002505e-11, "heading"=357.98244081345024}, {"position"=497.5857287577514, "velocity"=11.456511141170708, "acceleration"=-20.000000000000107, "jerk"=-1.7763568394002505e-11, "heading"=358.0524425224477}, {"position"=497.6992938691631, "velocity"=11.256511141170709, "acceleration"=-19.99999999999993, "jerk"=1.7763568394002505e-11, "heading"=358.1210072823765}, {"position"=497.81085898057484, "velocity"=11.05651114117071, "acceleration"=-19.99999999999993, "jerk"=0.0, "heading"=358.18814789291264}, {"position"=497.92042409198655, "velocity"=10.856511141170706, "acceleration"=-20.000000000000284, "jerk"=-3.552713678800501e-11, "heading"=358.25387693776474}, {"position"=498.02798920339825, "velocity"=10.656511141170707, "acceleration"=-19.99999999999993, "jerk"=3.552713678800501e-11, "heading"=358.3182067875358}, {"position"=498.13355431480994, "velocity"=10.456511141170706, "acceleration"=-20.000000000000107, "jerk"=-1.7763568394002505e-11, "heading"=358.38114960255507}, {"position"=498.2371194262216, "velocity"=10.256511141170707, "acceleration"=-19.99999999999993, "jerk"=1.7763568394002505e-11, "heading"=358.4427173356799}, {"position"=498.33868453763336, "velocity"=10.056511141170706, "acceleration"=-20.000000000000107, "jerk"=-1.7763568394002505e-11, "heading"=358.5029135092822}, {"position"=498.4382496490451, "velocity"=9.856511141170706, "acceleration"=-19.99999999999993, "jerk"=1.7763568394002505e-11, "heading"=358.5617530717863}, {"position"=498.5358147604568, "velocity"=9.656511141170707, "acceleration"=-19.99999999999993, "jerk"=0.0, "heading"=358.6192506796706}, {"position"=498.6313798718685, "velocity"=9.456511141170704, "acceleration"=-20.000000000000284, "jerk"=-3.552713678800501e-11, "heading"=358.6754174941808}, {"position"=498.7249449832802, "velocity"=9.256511141170705, "acceleration"=-19.99999999999993, "jerk"=3.552713678800501e-11, "heading"=358.73026448229683}, {"position"=498.81651009469186, "velocity"=9.056511141170702, "acceleration"=-20.000000000000284, "jerk"=-3.552713678800501e-11, "heading"=358.78380013176803}, {"position"=498.9060752061036, "velocity"=8.856511141170705, "acceleration"=-19.99999999999975, "jerk"=5.3290705182007514e-11, "heading"=358.83601895899795}, {"position"=498.9936403175153, "velocity"=8.656511141170704, "acceleration"=-20.000000000000107, "jerk"=-3.552713678800501e-11, "heading"=358.8869482593275}, {"position"=499.079205428927, "velocity"=8.456511141170704, "acceleration"=-19.99999999999993, "jerk"=1.7763568394002505e-11, "heading"=358.93659825771863}, {"position"=499.1627705403387, "velocity"=8.256511141170703, "acceleration"=-20.000000000000107, "jerk"=-1.7763568394002505e-11, "heading"=358.98497115523065}, {"position"=499.2443356517504, "velocity"=8.056511141170702, "acceleration"=-20.000000000000107, "jerk"=0.0, "heading"=359.0320659357662}, {"position"=499.3239007631621, "velocity"=7.856511141170704, "acceleration"=-19.99999999999984, "jerk"=2.6645352591003757e-11, "heading"=359.07790958216884}, {"position"=499.40146587457383, "velocity"=7.656511141170704, "acceleration"=-20.000000000000018, "jerk"=-1.7763568394002505e-11, "heading"=359.12250525838806}, {"position"=499.47703098598555, "velocity"=7.4565111411707, "acceleration"=-20.000000000000373, "jerk"=-3.552713678800501e-11, "heading"=359.165844084876}, {"position"=499.55059609739726, "velocity"=7.2565111411707, "acceleration"=-20.000000000000018, "jerk"=3.552713678800501e-11, "heading"=359.2079584205677}, {"position"=499.62216120880896, "velocity"=7.0565111411707, "acceleration"=-19.99999999999993, "jerk"=8.881784197001252e-12, "heading"=359.24883905622096}, {"position"=499.69172632022065, "velocity"=6.8565111411707, "acceleration"=-20.000000000000018, "jerk"=-8.881784197001252e-12, "heading"=359.28849605145274}, {"position"=499.75929143163233, "velocity"=6.656511141170701, "acceleration"=-19.99999999999993, "jerk"=8.881784197001252e-12, "heading"=359.32694861442155}, {"position"=499.82485654304406, "velocity"=6.456511141170701, "acceleration"=-20.000000000000018, "jerk"=-8.881784197001252e-12, "heading"=359.36417739278954}, {"position"=499.8884216544558, "velocity"=6.2565111411707, "acceleration"=-20.000000000000107, "jerk"=-8.881784197001252e-12, "heading"=359.4002223894028}, {"position"=499.9499867658675, "velocity"=6.0565111411707, "acceleration"=-19.99999999999993, "jerk"=1.7763568394002505e-11, "heading"=359.4350529696959}, {"position"=500.0095518772792, "velocity"=5.856511141170699, "acceleration"=-20.000000000000107, "jerk"=-1.7763568394002505e-11, "heading"=359.4687125939335}, {"position"=500.0671169886909, "velocity"=5.656511141170699, "acceleration"=-20.000000000000018, "jerk"=8.881784197001252e-12, "heading"=359.50117099144535}, {"position"=500.12268210010257, "velocity"=5.456511141170699, "acceleration"=-20.000000000000018, "jerk"=0.0, "heading"=359.53247047477106}, {"position"=500.1762472115143, "velocity"=5.2565111411707, "acceleration"=-19.99999999999993, "jerk"=8.881784197001252e-12, "heading"=359.5625773945708}, {"position"=500.227812322926, "velocity"=5.0565111411706996, "acceleration"=-20.000000000000018, "jerk"=-8.881784197001252e-12, "heading"=359.5915325162132}, {"position"=500.2773774343377, "velocity"=4.856511141170699, "acceleration"=-20.000000000000018, "jerk"=0.0, "heading"=359.61931588453973}, {"position"=500.3249425457494, "velocity"=4.656511141170699, "acceleration"=-20.000000000000018, "jerk"=0.0, "heading"=359.6459448321557}, {"position"=500.3705076571611, "velocity"=4.456511141170699, "acceleration"=-20.000000000000018, "jerk"=0.0, "heading"=359.6714279760057}, {"position"=500.4140727685728, "velocity"=4.2565111411707, "acceleration"=-19.99999999999993, "jerk"=8.881784197001252e-12, "heading"=359.69574787650197}, {"position"=500.4556378799845, "velocity"=4.0565111411706996, "acceleration"=-20.000000000000018, "jerk"=-8.881784197001252e-12, "heading"=359.71893394685014}, {"position"=500.49520299139624, "velocity"=3.856511141170699, "acceleration"=-20.00000000000006, "jerk"=-4.263256414560601e-12, "heading"=359.74097996765266}, {"position"=500.53276810280795, "velocity"=3.6565111411706996, "acceleration"=-19.99999999999993, "jerk"=1.3145040611561853e-11, "heading"=359.76187930093204}, {"position"=500.56833321421965, "velocity"=3.4565111411706995, "acceleration"=-20.000000000000018, "jerk"=-8.881784197001252e-12, "heading"=359.7816532399354}, {"position"=500.60190472105177, "velocity"=3.257790225253914, "acceleration"=-19.87209159167853, "jerk"=12.790840832148831, "heading"=359.80030742629623}, {"position"=500.6335184304894, "velocity"=3.0649516622783057, "acceleration"=-19.283856297560842, "jerk"=58.82352941176876, "heading"=359.81784220739314}, {"position"=500.663233166062, "velocity"=2.877995452243873, "acceleration"=-18.695621003443286, "jerk"=58.823529411755615, "heading"=359.83431428752914}, {"position"=500.691107751299, "velocity"=2.6969215951506174, "acceleration"=-18.107385709325552, "jerk"=58.82352941177338, "heading"=359.84975849696707}, {"position"=500.71720100972976, "velocity"=2.521730090998538, "acceleration"=-17.51915041520795, "jerk"=58.823529411760234, "heading"=359.8642089030049}, {"position"=500.7415717648837, "velocity"=2.3524209397876352, "acceleration"=-16.930915121090262, "jerk"=58.82352941176876, "heading"=359.87768636147456}, {"position"=500.7642788402902, "velocity"=2.188994141517908, "acceleration"=-16.342679826972706, "jerk"=58.823529411755615, "heading"=359.89023494093186}, {"position"=500.78538105947877, "velocity"=2.0314496961893584, "acceleration"=-15.754444532854972, "jerk"=58.82352941177338, "heading"=359.9018921563495}, {"position"=500.80493724597875, "velocity"=1.8797876038019847, "acceleration"=-15.166209238737371, "jerk"=58.823529411760056, "heading"=359.9126914703821}, {"position"=500.8230062233195, "velocity"=1.7340078643557877, "acceleration"=-14.577973944619703, "jerk"=58.823529411766806, "heading"=359.9226662294223}, {"position"=500.83964681503056, "velocity"=1.594110477850767, "acceleration"=-13.989738650502058, "jerk"=58.8235294117645, "heading"=359.9318496723611}, {"position"=500.85491784464125, "velocity"=1.4600954442869232, "acceleration"=-13.401503356384392, "jerk"=58.82352941176663, "heading"=359.9402667024542}, {"position"=500.86887813568103, "velocity"=1.3319627636642557, "acceleration"=-12.813268062266747, "jerk"=58.8235294117645, "heading"=359.94795714783965}, {"position"=500.88158651167925, "velocity"=1.2097124359827645, "acceleration"=-12.225032768149124, "jerk"=58.823529411762365, "heading"=359.95495630448585}, {"position"=500.89310179616535, "velocity"=1.0933444612424497, "acceleration"=-11.636797474031479, "jerk"=58.8235294117645, "heading"=359.9612970198354}, {"position"=500.90348281266876, "velocity"=0.9828588394433114, "acceleration"=-11.048562179913823, "jerk"=58.82352941176556, "heading"=359.96701207251334}, {"position"=500.9127883847189, "velocity"=0.8782555705853496, "acceleration"=-10.460326885796178, "jerk"=58.8235294117645, "heading"=359.9721341789699}, {"position"=500.92107733584515, "velocity"=0.7795346546685644, "acceleration"=-9.872091591678522, "jerk"=58.82352941176556, "heading"=359.9766959997789}, {"position"=500.92840848957695, "velocity"=0.6866960916929555, "acceleration"=-9.283856297560888, "jerk"=58.82352941176343, "heading"=359.9807301455967}, {"position"=500.9348406694437, "velocity"=0.5997398816585233, "acceleration"=-8.695621003443222, "jerk"=58.82352941176663, "heading"=359.98426918277914}, {"position"=500.9404326989748, "velocity"=0.5186660245652674, "acceleration"=-8.107385709325587, "jerk"=58.82352941176343, "heading"=359.9873456386608}, {"position"=500.9452434016997, "velocity"=0.44347452041318797, "acceleration"=-7.519150415207948, "jerk"=58.823529411763964, "heading"=359.9899920064959}, {"position"=500.9493316011478, "velocity"=0.3741653692022851, "acceleration"=-6.930915121090286, "jerk"=58.82352941176618, "heading"=359.9922407500619}, {"position"=500.95275612084845, "velocity"=0.3107385709325586, "acceleration"=-6.3426798269726525, "jerk"=58.82352941176334, "heading"=359.9941243079269}, {"position"=500.95557578433113, "velocity"=0.25319412560400867, "acceleration"=-5.754444532854991, "jerk"=58.82352941176618, "heading"=359.9956750973817}, {"position"=500.9578494151252, "velocity"=0.20153203321663513, "acceleration"=-5.166209238737355, "jerk"=58.82352941176361, "heading"=359.9969255180363}, {"position"=500.9596358367602, "velocity"=0.1557522937704381, "acceleration"=-4.577973944619703, "jerk"=58.823529411765115, "heading"=359.9979079550823}, {"position"=500.96099387276536, "velocity"=0.11585490726541754, "acceleration"=-3.9897386505020545, "jerk"=58.823529411764895, "heading"=359.99865478222017}, {"position"=500.9619823466702, "velocity"=0.08183987370157345, "acceleration"=-3.4015033563844095, "jerk"=58.8235294117645, "heading"=359.99919836425386}, {"position"=500.9626600820041, "velocity"=0.05370719307890581, "acceleration"=-2.813268062266763, "jerk"=58.82352941176463, "heading"=359.99957105935067}, {"position"=500.9630859022965, "velocity"=0.03145686539741465, "acceleration"=-2.225032768149116, "jerk"=58.82352941176472, "heading"=359.9998052209681}, {"position"=500.96331863107673, "velocity"=0.015088890657099964, "acceleration"=-1.6367974740314684, "jerk"=58.82352941176476, "heading"=359.9999331994473}, {"position"=500.9634170918743, "velocity"=0.0046032688579617466, "acceleration"=-1.0485621799138218, "jerk"=58.82352941176465, "heading"=359.99998734327335}, {"position"=500.9634401082186, "velocity"=0.0, "acceleration"=-0.46032688579617465, "jerk"=58.82352941176472, "heading"=6.3611093629270335e-15}, {"position"=500.9634401082186, "velocity"=0.0, "acceleration"=0.0, "jerk"=46.032688579617464, "heading"=6.3611093629270335e-15}]
  out "Position":cluster{dbl[], dbl[]}[](graph)
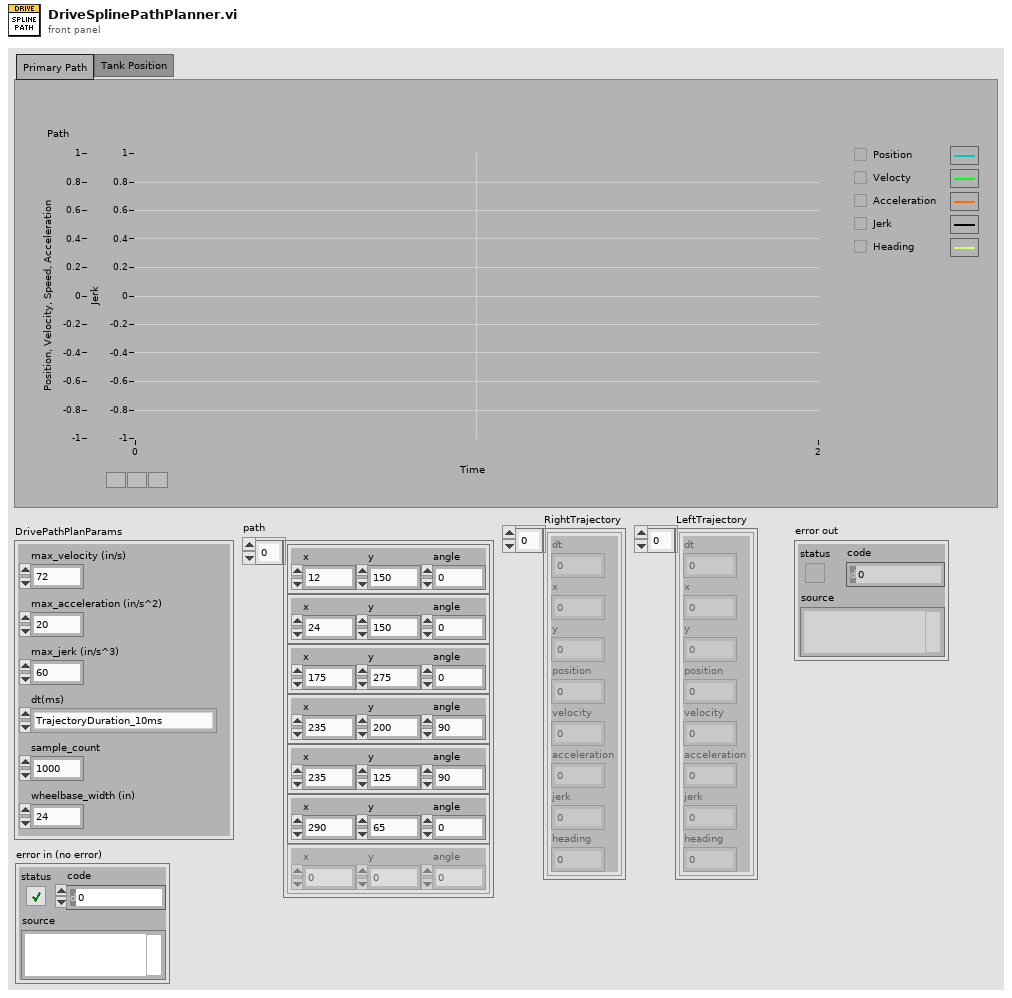
[diagram p1: front panel]
types:
  T1 = typedef "Pathfinder.lvlib/Segment.ctl" = cluster{"dt":dbl, "x":dbl, "y":dbl, "position":dbl, "velocity":dbl, "acceleration":dbl, "jerk":dbl, "heading":dbl}
  T2 = typedef "DrivePathfinderParams.ctl" = cluster{"max_velocity (in/s)":dbl, "max_acceleration (in/s^2)":dbl, "max_jerk (in/s^3)":dbl, "dt(ms)":T3, "sample_count":i32, "wheelbase_width (in)":dbl}
  T3 = typedef "CTRE_Phoenix_MotorControl_TrajectoryPointTimeDur.ctl" = i32
  T4 = cluster{"position":dbl, "velocity":dbl, "acceleration":dbl, "jerk":dbl, "heading":dbl}[]
  T5 = typedef "Pathfinder.lvlib/Waypoint.ctl" = cluster{"x":dbl, "y":dbl, "angle":dbl}
  T6 = cluster{"position":dbl, "velocity":dbl, "acceleration":dbl, "jerk":dbl, "heading":dbl}
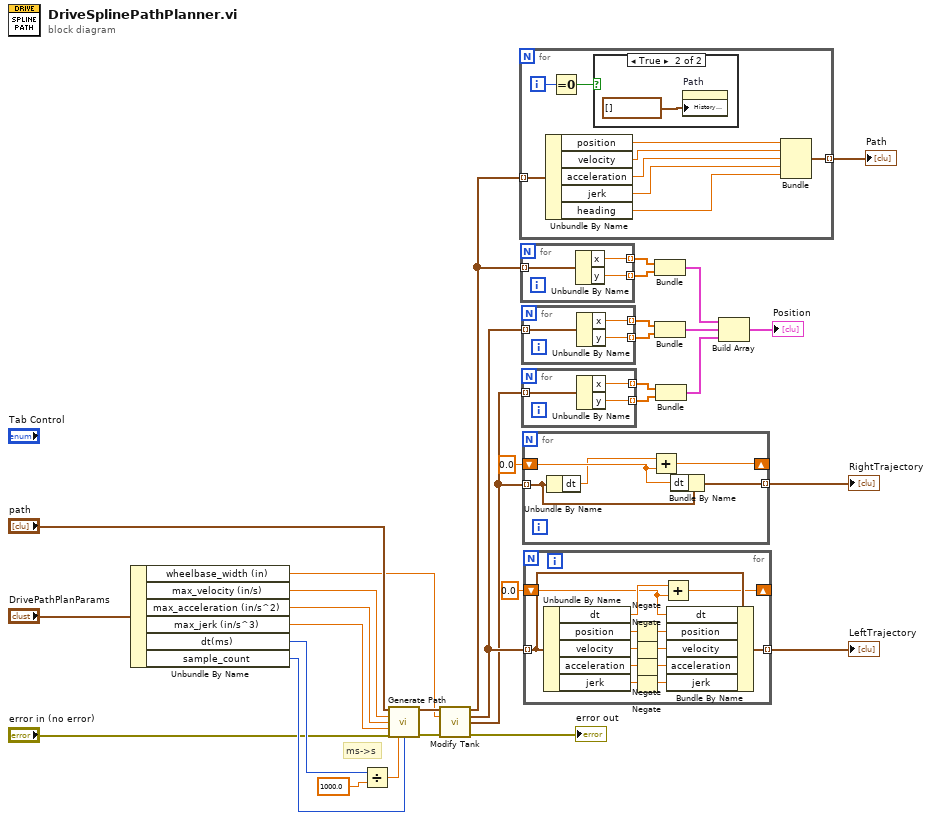
[diagram p0: block diagram]
diagram:
  # "ms->s"
  n1 = Unbundle By Name("DrivePathPlanParams") -> ("wheelbase_width (in)"=w11:dbl, "max_velocity (in/s)"=w10:dbl, "max_acceleration (in/s^2)"=w9:dbl, "max_jerk (in/s^3)"=w8:dbl, "dt(ms)"=w12:T3, "sample_count"=w13:i32)
  n2 = Divide(x=w12, y=1000.0) -> (x/y=w16:dbl)
  n3 = call "Generate Path.vi"("path"="path", "max_velocity"=w10, "max_acceleration"=w9, "max_jerk"=w8, "error in"="error in (no error)", "dt (.001)"=w16, "sample_count (100000)"=w13) -> ("Segments"=w32:T1[], "error out"=w30:errorcluster)  [unwired: 7 in]
  n4 = call "Modify Tank.vi"("Original"=w32, "wheelbase_width"=w11, "error in"=w30) -> ("original"=w21:T1[], "left"=w4:T1[], "right"=w1:T1[], "error out"=→"error out":errorcluster)  [unwired: 9 in]
  n5 = for {
    tunnel: w21 -> [w41] mode=indexing
    tunnel: [w35] -> w29 mode=indexing
    i -> [w34]
    n6 = Unbundle By Name(w41) -> ("position"=w40:dbl, "velocity"=w39:dbl, "acceleration"=w38:dbl, "jerk"=w37:dbl, "heading"=w36:dbl)
    n7 = Equal To 0?(x=w34) -> (x = 0?=w33:bool)
    n8 = case shown="True" w33 {
      frame False {
      }
      frame True {
        n9 = property on="Path" class="WFChart (strict)"("History Data"=T4 []) -> ()  [unwired: 2 in, 2 out]
      }
    }
    n10 = Bundle("position"=w40, "velocity"=w39, "acceleration"=w38, "jerk"=w37, "heading"=w36) -> (w35:T6)  [unwired: 1 in]
  }
  "Path" <- w29
  n11 = for {
    tunnel: w21 -> [w45] mode=indexing
    tunnel: [w44] -> w20 mode=indexing
    tunnel: [w43] -> w19 mode=indexing
    n12 = Unbundle By Name(w45) -> ("x"=w44:dbl, "y"=w43:dbl)
  }
  n13 = for {
    tunnel: w4 -> [w48] mode=indexing
    tunnel: [w47] -> w28 mode=indexing
    tunnel: [w46] -> w27 mode=indexing
    n14 = Unbundle By Name(w48) -> ("x"=w47:dbl, "y"=w46:dbl)
  }
  n15 = for {
    tunnel: w1 -> [w51] mode=indexing
    tunnel: [w50] -> w26 mode=indexing
    tunnel: [w49] -> w25 mode=indexing
    n16 = Unbundle By Name(w51) -> ("x"=w50:dbl, "y"=w49:dbl)
  }
  n17 = for {
    tunnel: w1 -> [w55] mode=indexing
    shift-right: [w56] -> _
    shift-left: 0.0 -> [w54]
    tunnel: [w52] -> w2 mode=indexing
    n18 = Unbundle By Name(w55) -> ("dt"=w53:dbl)
    n19 = Add(x=w53, y=w54) -> (x+y=w56:dbl)
    n20 = Bundle By Name(cluster=w55, "dt"=w54) -> (w52:T1)
  }
  "RightTrajectory" <- w2
  n21 = for {
    tunnel: w4 -> [w64] mode=indexing
    tunnel: [w67] -> w3 mode=indexing
    shift-right: [w59] -> _
    shift-left: 0.0 -> [w57]
    n22 = Unbundle By Name(w64) -> ("dt"=w58:dbl, "position"=w69:dbl, "velocity"=w68:dbl, "acceleration"=w63:dbl, "jerk"=w62:dbl)
    n23 = Negate(x=w69) -> (-x=w66:dbl)
    n24 = Negate(x=w68) -> (-x=w65:dbl)
    n25 = Negate(x=w63) -> (-x=w61:dbl)
    n26 = Negate(x=w62) -> (-x=w60:dbl)
    n27 = Add(x=w58, y=w57) -> (x+y=w59:dbl)
    n28 = Bundle By Name(cluster=w64, "dt"=w57, "position"=w66, "velocity"=w65, "acceleration"=w61, "jerk"=w60) -> (w67:T1)
  }
  "LeftTrajectory" <- w3
  n29 = Bundle(w20, w19) -> (w18:cluster{dbl[], dbl[]})  [unwired: 1 in]
  n30 = Bundle(w28, w27) -> (w23:cluster{dbl[], dbl[]})  [unwired: 1 in]
  n31 = Bundle(w26, w25) -> (w24:cluster{dbl[], dbl[]})  [unwired: 1 in]
  n32 = Build Array(w18, w23, w24) -> (→"Position":cluster{dbl[], dbl[]}[])
